vi "Process.vi"(8 "error in":errorcluster, 11 "Inst.Attocube-3DR":refnum<class "Inst.Attocube-3DR.lvclass">) -> (0 "error out":errorcluster, 3 "Inst.Attocube-3DR out":refnum<class "Inst.Attocube-3DR.lvclass">)   [LabVIEW 2019, in "Inst.Attocube-3DR.lvclass"]
doc: "---------------------------------------------------------------\nJKI State Machine Objects™\nhttp://jki.net/state-machine-objects/\nCopyright (C) 2005-2015, JKI <info@jki.net>\nALL RIGHTS RESERVED"
uses:
  Inst.Attocube-3DR.lvclass
  <vilib>/JKI/JKI SMO/SMO/SMO.lvclass
  <userlib>/LevyLab/Instrument Framework/SMOs/Instrument/Instrument.lvclass
  C:/Program Files (x86)/National Instruments/LabVIEW 2019/user.lib/LevyLab/Instrument Framework/Instrument Types/VSource/Instrument.VSource.lvclass
  C:/Program Files (x86)/National Instruments/LabVIEW 2019/user.lib/LevyLab/Instrument Framework/SMOs/Instrument/Instrument.lvclass
  C:/Program Files (x86)/National Instruments/LabVIEW 2019/vi.lib/JKI/JKI SMO/SMO/SMO.lvclass
  <userlib>/LevyLab/Instrument Framework/SMOs/RemoteControl/Typedefs/Message--Cluster.ctl
  <userlib>/LevyLab/Instrument Framework/SMOs/RemoteControl/RemoteControl.lvclass
  Typedefs/PrivateEvents--Inst.Attocube-3DR.MessageToProcess.ctl
  <userlib>/LevyLab/Instrument Framework/Instrument Types/VSource/Instrument.VSource.lvclass
  02efe66c-2260-4f62-810d-420fe48266f6.vi
  Typedefs/Inst.Attocube-3DR.Inputs--Cluster.ctl
  b2d5f30b-306e-4431-881a-eae28691b89f.vi
  0d401355-90ab-4fe7-b69d-5d5dba6cf2d1.vi
  f6063e37-5151-4c3e-a0a1-ff20a9429030.vi
  b7011c9a-a6eb-4fed-9c65-84cbf090edec.vi
  a7b2e31e-1869-440d-b8a6-16844ca516c9.vi
  646a4127-2411-415a-a65c-d25643f6d308.vi
  9e0d4248-952c-4312-a65b-c2252510a20b.vi
  91b4fc71-810e-4ac6-861b-a834e2ae1df3.vi
  7463a076-c03a-4db0-a820-c31f80c245ec.vi
  b30ad2a8-5df5-4a5a-98b2-da7e262b1587.vi
  0967008a-f394-440b-b6da-68de688ceb32.vi
  53937d0e-537d-4a87-94d7-f09408c92319.vi
  61d2fe89-1505-4e67-8cee-d03c7fbfaeb2.vi
panel:
  out "Status":string
  out "State History":string
  # "Instrument.Framework-Template"
  # "Framework-Template"
  # "For instructions on how to use the JKI State Machine Objects, examples and video tutorials, visit:\nhttp://jki.net/state-machine-objects/\n\nJKI State Machine Objects™\nhttp://jki.net/state-machine-objects/\nCopyright (C) 2005-2015, JKI <info@jki.net>\nALL RIGHTS RESERVED"
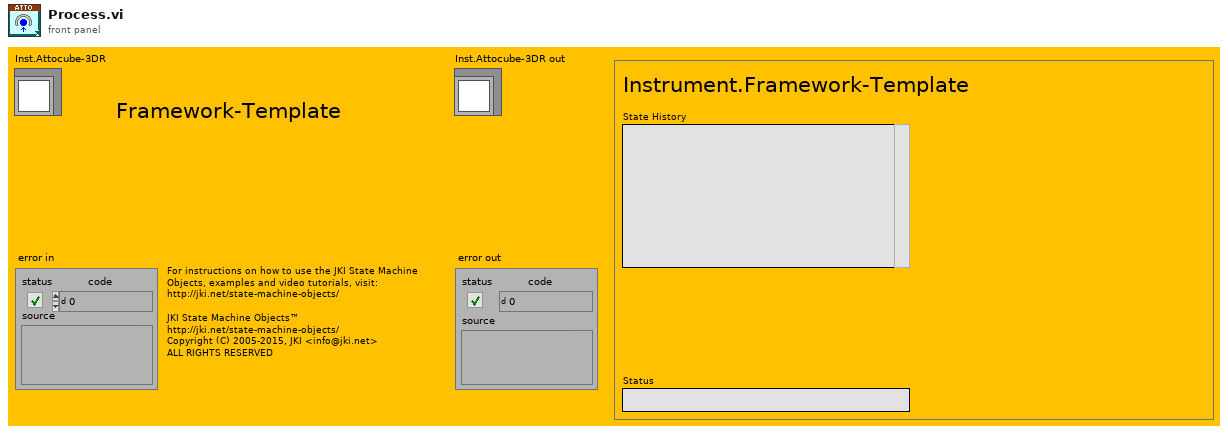
[diagram p1: front panel]
types:
  T1 = enum32{"invalid app kind", "Development System", "Run Time System", "Student Edition", "Embedded LabVIEW", "Evaluation", "Custom"}
  T2 = enum32{"Invalid", "Standard", "Closed", "Hidden", "Minimized", "Maximized"}
  T3 = typedef "RemoteControl.lvclass/Message--Cluster.ctl" = cluster{"Command":string, "Data":variant, "ID":string}
  T4 = typedef "Inst.Attocube-3DR.lvclass/PrivateEvents--Inst.Attocube-3DR.MessageToProcess.ctl" = cluster{"Message":T3}
  T5 = cluster{"Core":cluster{"Current VI Reference":refnum<vi>, "Close Panel on Exit?":bool, "Last Error":cluster{"error":errorcluster, "previous state":string, "remaining states":string}, "Shutdown?":bool}, "SelfRef":refnum<class "Inst.Attocube-3DR.lvclass">, "Running Step":i32, "sequence":string[], "MessageToProcess":T4}
  T6 = cluster{"Current VI Reference":refnum<vi>, "Close Panel on Exit?":bool, "Last Error":cluster{"error":errorcluster, "previous state":string, "remaining states":string}, "Shutdown?":bool}
  T7 = typedef "SMO.lvclass/Protected Events.ctl" = cluster{"StopProcesses":refnum<user-event>, "AbortProcesses":refnum<user-event>, "Config Changed":refnum<user-event>, "Dependency":refnum<user-event>}
  T8 = typedef "Inst.Attocube-3DR.lvclass/Inst.Attocube-3DR.Inputs--Cluster.ctl" = cluster{"Handle":i32, "Axes Number":u8, "Axis 1: sp Position":dbl, "Axis 2: sp Position":dbl, "Axis 1: sp rot count":i32, "Axis 2: sp rot count":i32, "Backward or Forward?":bool, "Axis 1: Amplitude [V] ":dbl, "Axis 2: Amplitude [V] ":dbl, "Axis 1: DCLevel [V]":dbl, "Axis 2: DCLevel [V]":dbl, "Axis 1: Frequency [Hz]":i32, "Axis 2: Frequency [Hz]":i32, "Axis 1:\ncontrol mode":enum16{"speed", "amplitude", "step size"}, "Axis 2:\ncontrol mode":enum16{"speed", "amplitude", "step size"}, "axis 1:\nOutput":bool, "axis 2:\nOutput 2":bool, "axis 1:\nstop detection":bool, "axis 2:\nstop detection":bool, "axis 1:\nSingle Circle Mode":bool, "axis 2:\nSingle Circle Mode":bool, "axis 1: \nTarget GND":bool, "axis 2: \nTarget GND":bool}
  T9 = cluster{"error ":bool, "error number":i32, "error code":string}
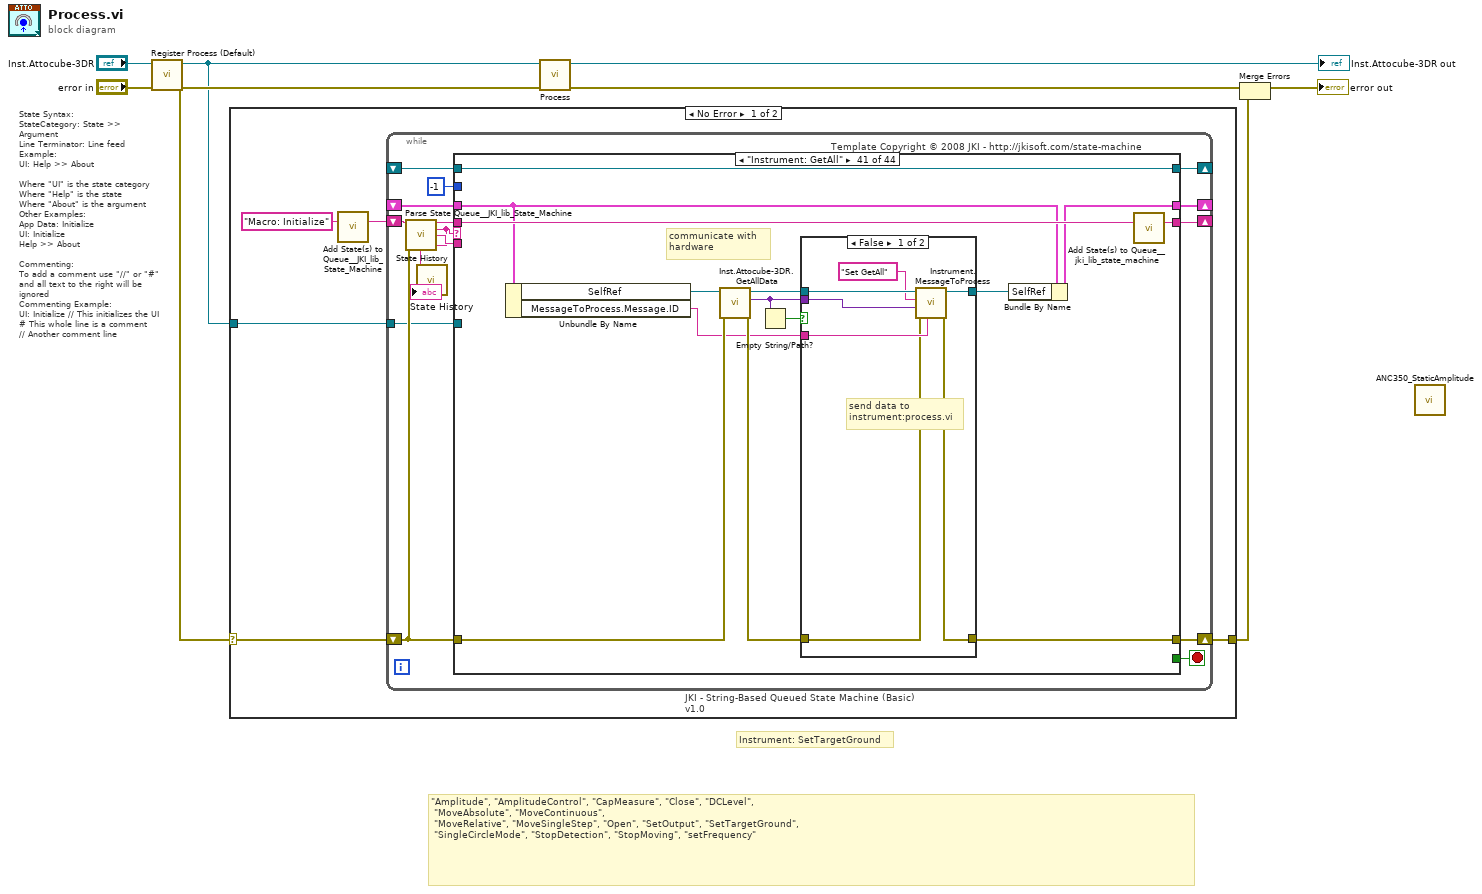
[diagram p0: block diagram]
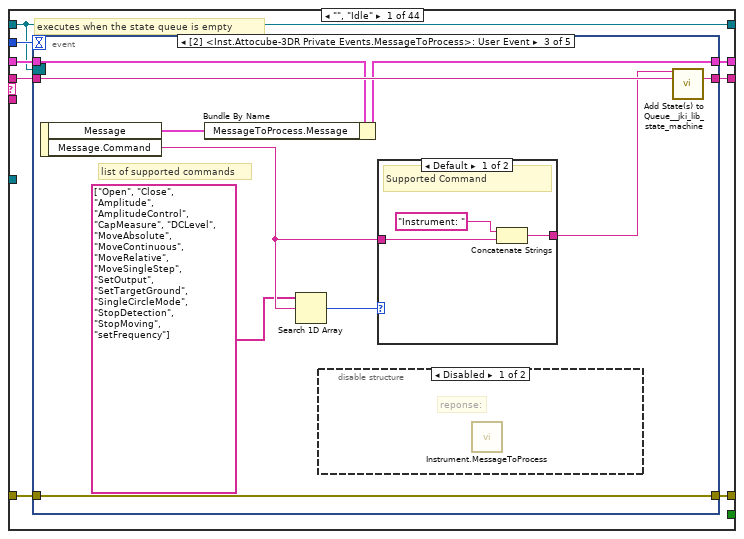
[diagram p2: hidden frame]
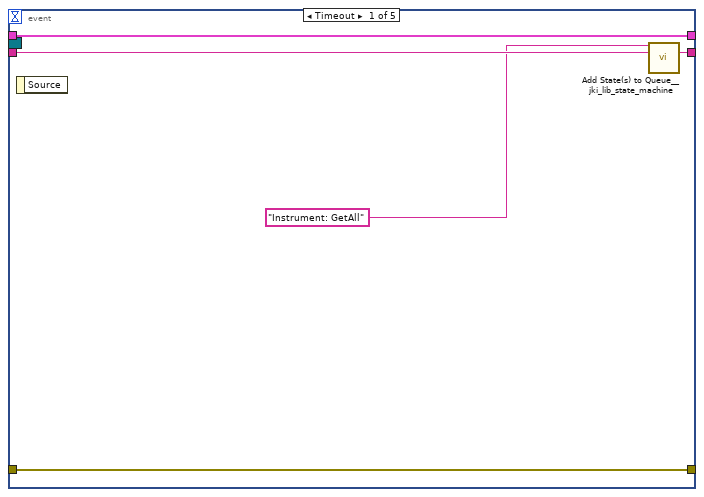
[diagram p3: hidden frame]
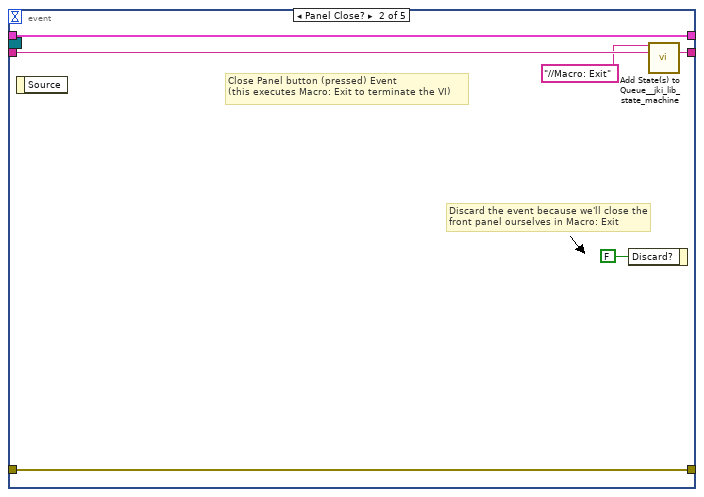
[diagram p4: hidden frame]
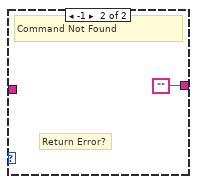
[diagram p6: hidden frame]
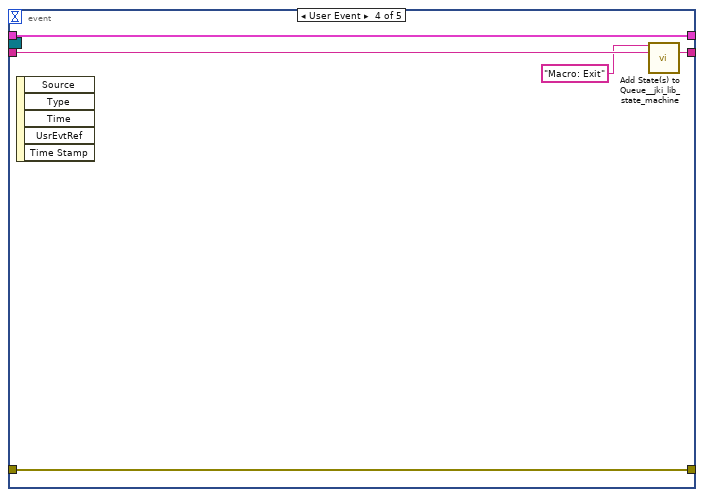
[diagram p7: hidden frame]
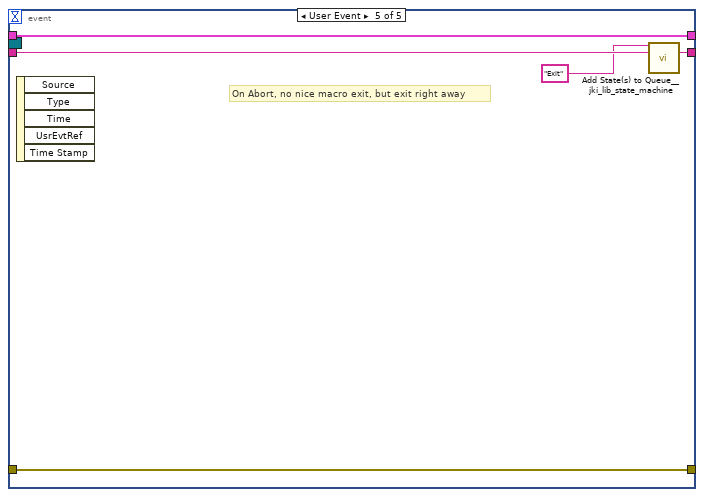
[diagram p8: hidden frame]
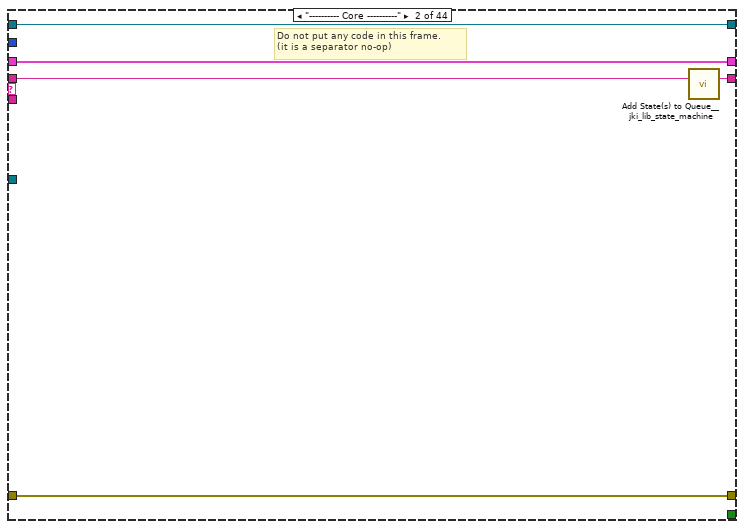
[diagram p9: hidden frame]
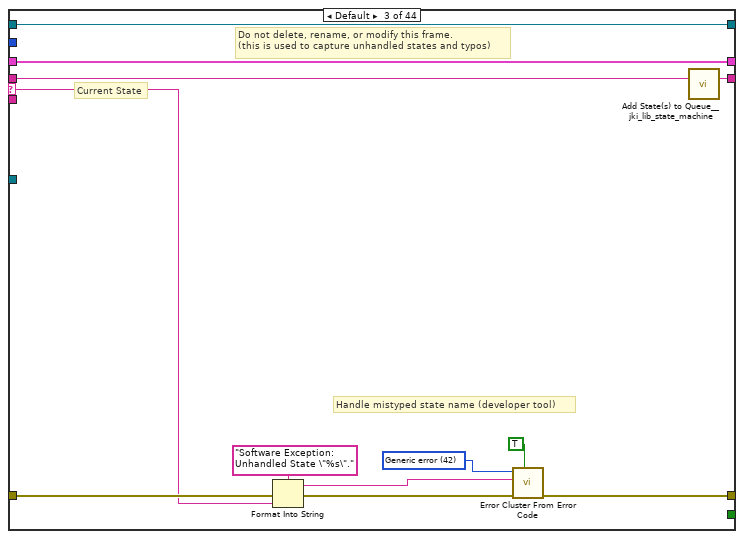
[diagram p10: hidden frame]
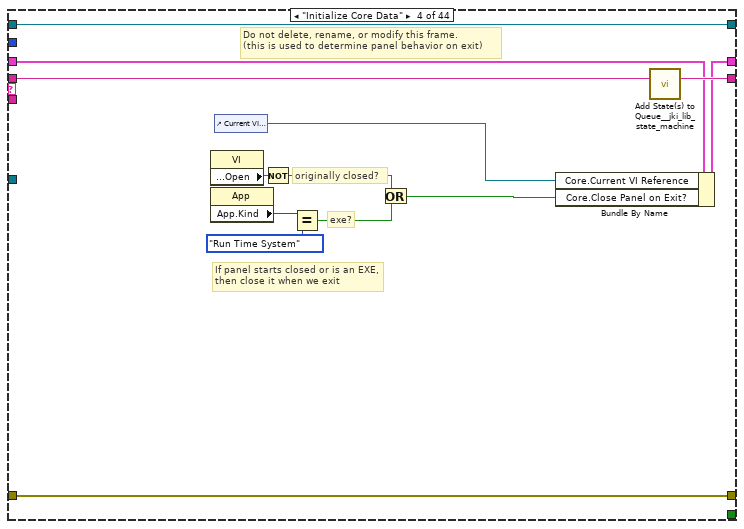
[diagram p11: hidden frame]
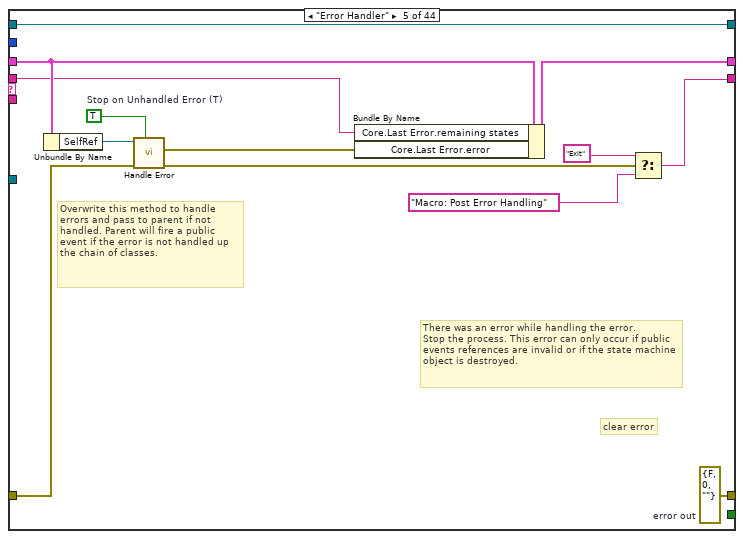
[diagram p12: hidden frame]
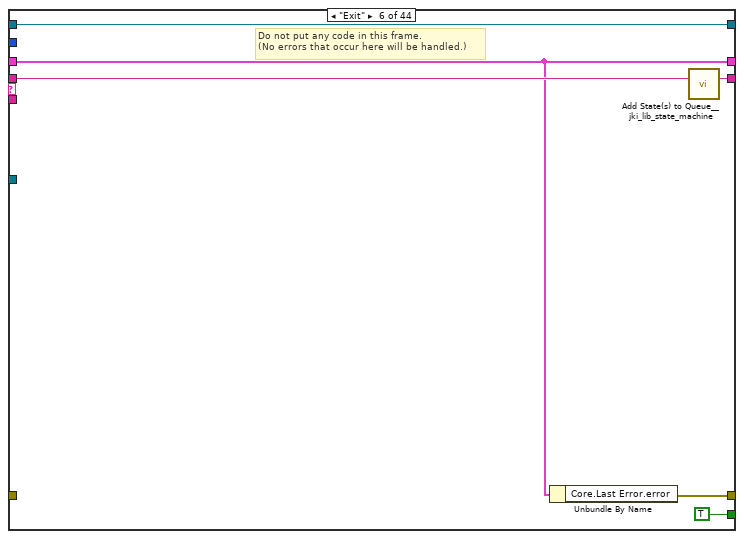
[diagram p13: hidden frame]
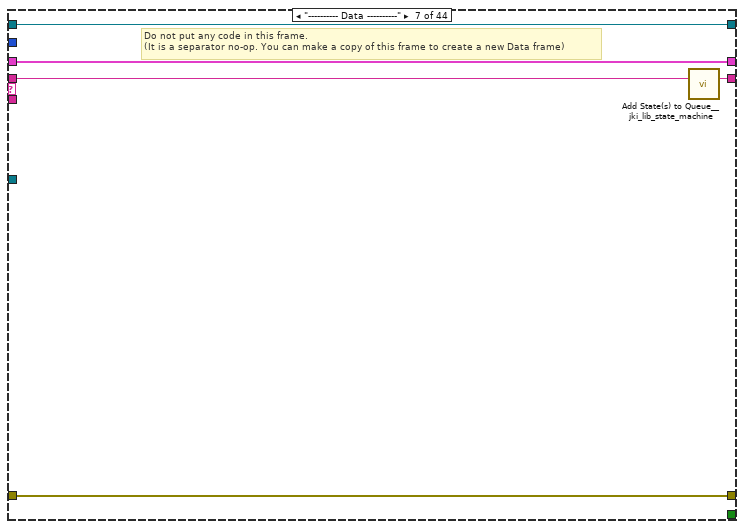
[diagram p14: hidden frame]
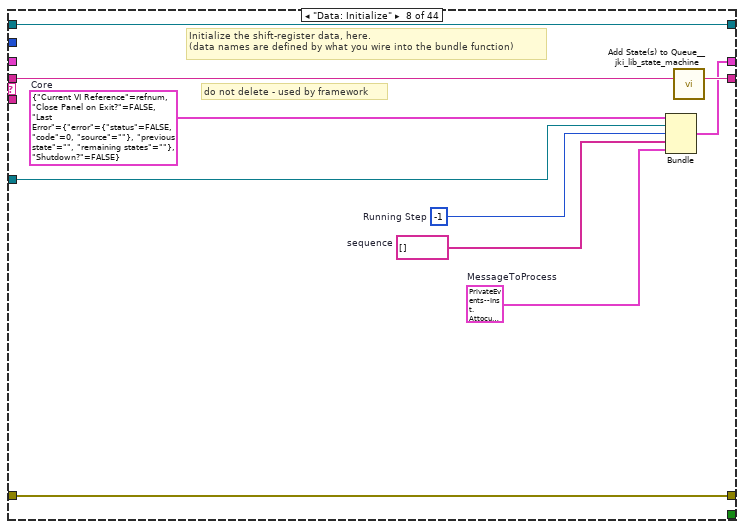
[diagram p15: hidden frame]
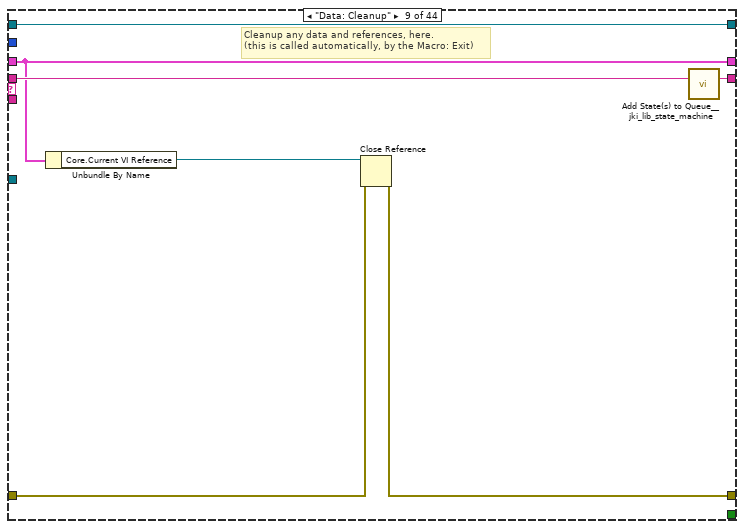
[diagram p16: hidden frame]
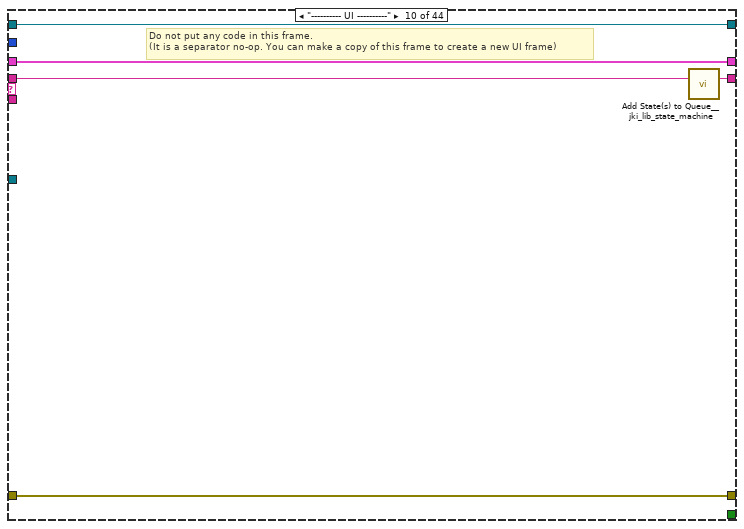
[diagram p17: hidden frame]
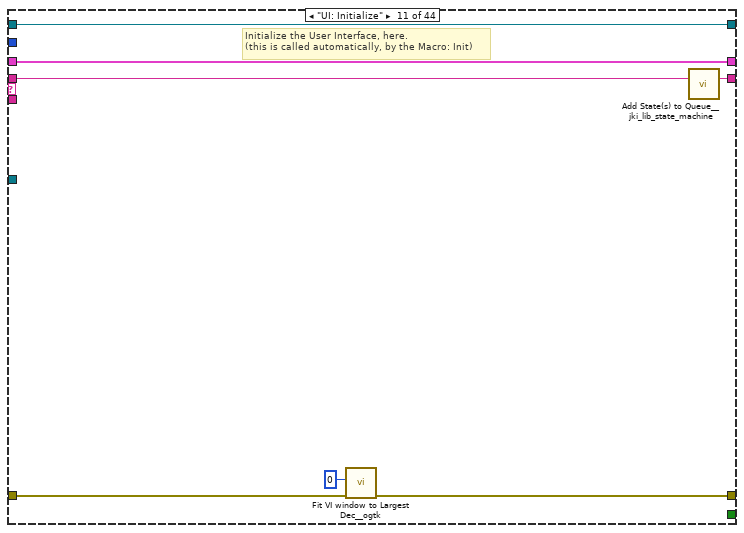
[diagram p18: hidden frame]
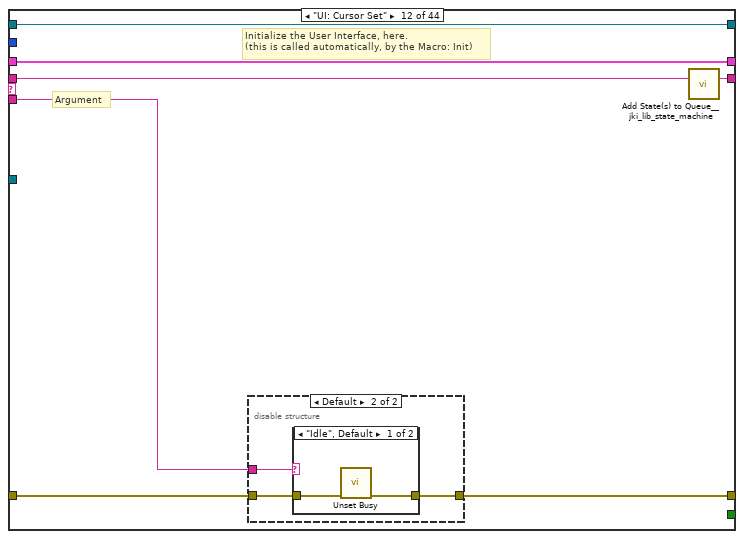
[diagram p19: hidden frame]
diagram:
  # "Instrument: SetTargetGround"
  # "\"Amplitude\", \"AmplitudeControl\", \"CapMeasure\", \"Close\", \"DCLevel\",\n \"MoveAbsolute\", \"MoveContinuous\",\n \"MoveRelative\", \"MoveSingleStep\", \"Open\", \"SetOutput\", \"SetTargetGround\",\n \"SingleCircleMode\", \"StopDetection\", \"StopMoving\", \"setFrequency\""
  # "State Syntax:\nStateCategory: State >> Argument\nLine Terminator: Line feed\nExample:\nUI: Help >> About\n\nWhere \"UI\" is the state category\nWhere \"Help\" is the state\nWhere \"About\" is the argument\nOther Examples:\nApp Data: Initialize\nUI: Initialize\nHelp >> About\n\nCommenting:\nTo add a comment use \"//\" or \"#\" and all text to the right will be ignored\nCommenting Example:\nUI: Initialize // This initializes the UI\n# This whole line is a comment\n// Another comment line"
  n1 = call <vilib>:"Register Process (Default).vi"("error in (no error)"="error in", "SMO"="Inst.Attocube-3DR") -> ("error out"=w5:errorcluster, "SelfRef"=w4:refnum<class "Inst.Attocube-3DR.lvclass">)  [unwired: 8 in]
  n2 = case shown="No Error" w5 {
    selector: w5 -> [w10 w732]
    tunnel: w4 -> [w11 _]
    tunnel: [w9 w732] -> w1
    frame No Error {
      n3 = call <vilib>:"Add State(s) to Queue__JKI_lib_State_Machine.vi"("State(s) in (\"\")"="Macro: Initialize") -> ("States Out"=w13:string)  [unwired: 14 in]
      n4 = while "JKI - String-Based Queued State Machine (Basic) v1.0" {
        shift-right: [w22] -> _
        shift-left: _ -> [w21]
        shift-right: [w25] -> w9
        shift-left: w10 -> [w19]
        shift-right: [w24] -> _
        shift-left: w13 -> [w26]
        tunnel: w11 -> [w18]
        shift-right: [w17] -> _
        shift-left: _ -> [w16]
        stop <- w23 stop-if-true
        # "Template Copyright © 2008 JKI - http://jkisoft.com/state-machine"
        n5 = call <vilib>:"Parse State Queue__JKI_lib_State_Machine.vi"("State Queue"=w26, "Error In (no error)"=w19) -> ("Remaining States"=w28:string, "Current State"=w15:string, "Arguments"=w27:string)  [unwired: 11 in]
        n6 = call <userlib>:"State History.vi"("Current State"=w15) -> ("History"=→"State History":string)  [unwired: 10 in]
        n7 = case shown="\"Instrument: GetAll\"" w15 {
          selector: w15 -> [_ _ w78 _ _ _ _ _ _ _ _ _ _ _ _ _ _ _ _ _ _ _ _ _ _ _ _ _ _ _ _ _ _ _ _ _ _ _ _ _ _ _ _ _]
          tunnel: w28 -> [w36 w76 w82 w101 w106 w120 w125 w135 w142 w147 w154 w161 w177 w209 w228 w240 w261 w283 w288 w299 w304 w317 w323 w330 w347 w369 w390 w413 w436 w459 w482 w505 w529 w555 w581 w608 w631 w654 w669 w678 w692 w706 w712 w731]
          tunnel: w27 -> [_ _ _ _ _ _ _ _ _ _ _ w155 w171 _ _ _ _ _ _ _ _ _ _ _ _ _ _ _ _ _ _ _ _ _ _ _ _ _ _ _ _ _ w707 w715]
          tunnel: w21 -> [w34 w73 w80 w92 w110 w116 w122 _ w137 w144 w152 w159 w173 w206 w225 w230 w251 w264 w285 w296 w301 w310 w321 w325 w343 w365 w386 w409 w432 w455 w478 w501 w525 w551 w577 w604 w627 w650 w665 w674 w680 w702 w708 w721]
          tunnel: [w33 w74 w84 w98 w111 w115 w123 w127 w138 w145 w149 w156 w174 w207 w213 w238 w259 w266 w286 w290 w302 w313 w319 w327 w332 w355 w374 w399 w420 w443 w470 w493 w513 w538 w566 w593 w615 w641 w662 w671 w685 w703 w709 w723] -> w25
          tunnel: w19 -> [w32 w74 w83 w98 w112 _ w123 w127 w139 w145 w148 w157 w175 w207 w217 w238 w259 w267 w286 w291 w302 w307 w319 w327 w333 w356 w375 w400 w421 w444 w469 w492 w514 w539 w567 w594 w616 w642 w661 w670 w688 w703 w709 w717]
          tunnel: [w35 w75 w81 w100 w102 w119 w124 w134 w141 w146 w153 w160 w176 w208 w227 w239 w260 w282 w287 w298 w303 w316 w322 w329 w346 w368 w389 w412 w435 w458 w481 w504 w528 w554 w580 w607 w630 w653 w668 w677 w691 w705 w711 w730] -> w24
          tunnel: [_ _ _ _ _ TRUE _ _ _ _ _ _ _ _ _ _ _ _ _ _ _ _ _ _ _ _ _ _ _ _ _ _ _ _ _ _ _ _ _ _ _ _ _ _] -> w23
          tunnel: [w31 w73 w80 w99 w109 w116 w122 w133 w137 w144 w152 w159 w173 w206 w225 w231 w252 w264 w285 w296 w301 w310 w321 w326 w344 w366 w387 w410 w433 w456 w479 w502 w526 w552 w578 w605 w628 w651 w666 w675 w689 w702 w708 w720] -> w22
          tunnel: -1 ("Timeout") -> [w30 _ _ _ _ _ _ _ _ _ _ _ _ _ _ _ _ _ _ _ _ _ _ _ _ _ _ _ _ _ _ _ _ _ _ _ _ _ _ _ _ _ _ _]
          tunnel: w18 -> [_ _ _ _ _ _ _ w128 _ _ _ _ _ _ w221 _ _ w263 _ _ _ _ _ _ _ _ _ _ _ _ _ _ _ _ _ _ _ _ _ _ _ _ _ _]
          tunnel: [w29 w72 w77 w89 w114 w117 w121 w132 w136 w143 w151 w158 w170 w205 w226 w237 w258 w277 w284 w297 w300 w315 w320 w328 w345 w367 w388 w411 w434 w457 w480 w503 w527 w553 w579 w606 w629 w652 w667 w676 w690 w704 w710 w729] -> w17
          tunnel: w16 -> [w29 w72 w77 w89 w114 w117 w121 w132 w136 w143 w151 w158 w170 w205 w226 w237 w258 w277 w284 w297 w300 _ w320 w328 w345 w367 w388 w411 w434 w457 w480 w503 w527 w553 w579 w606 w629 w652 w667 w676 w690 w704 w710 w729]
          frame "", "Idle" {
            # "executes when the state queue is empty"
            n8 = event shown="[2] <Inst.Attocube-3DR Private Events.MessageToProcess>: User Event" {
              selector: w29 -> [_ _ _ _ _]
              dyn-events: _ -> [_ _ _ _ _]
              timeout: w30 -> [_ _ _ _ _]
              tunnel: w36 -> [w41 w47 w57 w66 w71]
              tunnel: [w40 w46 w56 w65 w70] -> w35
              tunnel: w34 -> [w38 w44 w50 w63 w68]
              tunnel: [w39 w45 w55 w64 w69] -> w33
              tunnel: w32 -> [w39 w45 w55 w64 w69]
              tunnel: [w38 w44 w51 w63 w68] -> w31
              event Timeout {
                n9 = event-data() -> ()  [unwired: 1 in, 1 out]
                n10 = call <vilib>:"Add State(s) to Queue__jki_lib_state_machine.vi"("State(s) in Front (\"\")"="Instrument: GetAll" ("State(s) in Front (\"\")"), "State(s) in (\"\")"=w41) -> ("States Out"=w40:string)  [unwired: 13 in]
              }
              event Panel Close? {
                # "Discard the event because we'll close the front panel ourselves in Macro: Exit"
                # "Close Panel button (pressed) Event\n(this executes Macro: Exit to terminate the VI)"
                n11 = event-data() -> ()  [unwired: 1 in, 1 out]
                n12 = event-data("Discard?"=FALSE) -> ()  [unwired: 1 in, 1 out]
                n13 = call <vilib>:"Add State(s) to Queue__jki_lib_state_machine.vi"("State(s) in Front (\"\")"="//Macro: Exit", "State(s) in (\"\")"=w47) -> ("States Out"=w46:string)  [unwired: 13 in]
              }
              event User Event {
                # "list of supported commands"
                n14 = event-data() -> ("Message"=w49:T3, "Message.Command"=w52:string)  [unwired: 1 in]
                n15 = Bundle By Name(cluster=w50, "MessageToProcess.Message"=w49) -> (w51:T5)
                n16 = Search 1D Array(1D array=string[] ["Open", "Close", "Amplitude", "AmplitudeControl", "CapMeasure", "DCLevel", "MoveAbsolute", "MoveContinuous", "MoveRelative", "MoveSingleStep", "SetOutput", "SetTargetGround", "SingleCircleMode", "StopDetection", "StopMoving", "setFrequency"], element=w52) -> (index of element=w54:i32)  [unwired: 1 in]
                n17 = disable-structure shown="Disabled" {
                  frame Disabled {
                    # "reponse:"
                    n18 = call <userlib>:"Instrument.MessageToProcess.vi"() -> ()  [unwired: 10 in, 2 out]
                  }
                  frame Enabled {
                  }
                }
                n19 = case shown="Default" w54 {
                  tunnel: [w60 "" ("Empty String Constant")] -> w53
                  tunnel: w52 -> [w59 _]
                  frame Default {
                    # "Supported Command"
                    n20 = Concatenate Strings("Instrument: ", w59) -> (w60:string)
                  }
                  frame -1 {
                    # "Return Error?"
                    # "Command Not Found"
                  }
                }
                n21 = call <vilib>:"Add State(s) to Queue__jki_lib_state_machine.vi"("State(s) in Front (\"\")"=w53, "State(s) in (\"\")"=w57) -> ("States Out"=w56:string)  [unwired: 13 in]
              }
              event User Event {
                n22 = event-data() -> ()  [unwired: 1 in, 5 out]
                n23 = call <vilib>:"Add State(s) to Queue__jki_lib_state_machine.vi"("State(s) in Front (\"\")"="Macro: Exit", "State(s) in (\"\")"=w66) -> ("States Out"=w65:string)  [unwired: 13 in]
              }
              event User Event {
                # "On Abort, no nice macro exit, but exit right away"
                n24 = event-data() -> ()  [unwired: 1 in, 5 out]
                n25 = call <vilib>:"Add State(s) to Queue__jki_lib_state_machine.vi"("State(s) in Front (\"\")"="Exit", "State(s) in (\"\")"=w71) -> ("States Out"=w70:string)  [unwired: 13 in]
              }
            }
          }
          frame "---------- Core ----------" {
            # "Do not put any code in this frame.\n(it is a separator no-op)"
            n26 = call <vilib>:"Add State(s) to Queue__jki_lib_state_machine.vi"("State(s) in (\"\")"=w76) -> ("States Out"=w75:string)  [unwired: 14 in]
          }
          frame Default {
            w87 = 42 items=["No error", "Argument error", "Memory is full", "Out of zone", "End of file", "File already open", "Generic file I/O error", "File not found", "File permission error", "Disk is full", "Duplicate path", "Too many files open", "System feature not enabled", "Resource file not found", "Cannot add resource", "Resource not found", "Image not found", "Image memory error", "Pen does not exist", "Config type invalid", "Config token not found", "Config parse error", "Config memory error", "Bad external code format", "Bad external code offset", "External code not present", "Null window", "Destroy window error", "Null menu", "Print aborted", "Bad print record", "Print driver error", "Windows error during printing", "Memory error during printing", "Print dialog error", "Generic print error", "Invalid device refnum", "Device not found", "Device parameter error", "Device unit error", "Cannot open device", "Device call aborted", "Generic error", "Cancelled by user", "Object ID too low", "Object ID too high", "Object not in heap", "Unknown heap", "Unknown object (invalid DefProc)", "Unknown object (DefProc not in table)", "Message out of range", "Invalid (null) method", "Unknown message", "Manager call not supported", "Bad address", "Network operation in progress", "Network operation timed out", "Connection is busy", "Network attribute not supported", "Network error", "Address in use", "System out of memory", "Connection aborted", "Connection refused", "Not connected", "Already connected", "Connection closed", "Initialization error (interapplication manager)", "Bad occurrence", "Wait on unbound occurrence handler", "Occurrence queue overflow", "Datalog type conflict", "Unused", "Unrecognized type (interapplication manager)", "Memory corrupt", "Failed to make temporary DLL", "Old CIN version", "Drag socket not found", "Failed to load drop-object", "Failed to register OLE object", "Failed to release OLE object", "Format specifier type mismatch", "Unknown format specifier", "Too few format specifiers", "Too many format specifiers", "Scan failed", "Newer CIN version", "Error converting to variant", "Runtime menu error", "Password tampered", "Variant attribute not found", "Incompatible variant data type", "Event data is not available", "Event Store is not present", "Occurrence is not found", "Event Queue is not created", "Event info is not available", "Refnum passed is NULL", "Error retrieving Class GUID", "Error retrieving CoClass GUID", "Error retrieving TypeLib GUID.", "Bad built application magic bytes.", "Specific driver is different from the specific driver associated with the Logical Name.", "There is no session opened to the class driver.", "Max Error", "MAX - Error with config objects", "MAX - Error loading configuration", "MAX - Group not supported"]
            # "Current State"
            # "Do not delete, rename, or modify this frame.\n(this is used to capture unhandled states and typos)"
            # "Handle mistyped state name (developer tool)"
            n27 = Format Into String(format string="Software Exception: Unhandled State \"%s\"." ("message"), error in=w83, w78) -> (resulting string=w86:string, error out=w85:errorcluster)  [unwired: 1 in]
            n28 = call <vilib>:"Error Cluster From Error Code.vi"("show call chain? (False)"=TRUE, "error in (no error)"=w85, "error message (\"\")"=w86, "error code (0)"=w87) -> ("error out"=w84:errorcluster)  [unwired: 5 in]
            n29 = call <vilib>:"Add State(s) to Queue__jki_lib_state_machine.vi"("State(s) in (\"\")"=w82) -> ("States Out"=w81:string)  [unwired: 14 in]
          }
          frame "Initialize Core Data" {
            # "Do not delete, rename, or modify this frame.\n(this is used to determine panel behavior on exit)"
            # "originally closed?"
            # "exe?"
            # "If panel starts closed or is an EXE, then close it when we exit"
            n30 = property class="VI"() -> ("Front Panel.Open"=w97:bool)  [unwired: 2 in, 2 out]
            n31 = property class="App"() -> ("App.Kind"=w96:T1)  [unwired: 2 in, 2 out]
            n32 = control-ref of="Current VI Reference"() -> (w90:refnum<vi>)
            n33 = Not(x=w97) -> (.not. x?=w94:bool)
            n34 = Equal?(x=w96, y=T1."Run Time System" ("Application:Kind")) -> (x = y?=w93:bool)
            n35 = Or(x=w94, y=w93) -> (x .or. y?=w91:bool)
            n36 = Bundle By Name(cluster=w92, "Core.Current VI Reference"=w90, "Core.Close Panel on Exit?"=w91) -> (w99:T5)
            n37 = call <vilib>:"Add State(s) to Queue__jki_lib_state_machine.vi"("State(s) in (\"\")"=w101) -> ("States Out"=w100:string)  [unwired: 14 in]
          }
          frame "Error Handler" {
            w107 = TRUE  # Stop on Unhandled Error (T)
            w111 = errorcluster {"status"=FALSE, "code"=0, "source"=""}  # error out
            # "clear error"
            # "There was an error while handling the error.\nStop the process. This error can only occur if public events references are invalid or if the state machine object is destroyed."
            # "Overwrite this method to handle errors and pass to parent if not handled. Parent will fire a public event if the error is not handled up the chain of classes."
            n38 = Unbundle By Name(w110) -> ("SelfRef"=w113:refnum<class "Inst.Attocube-3DR.lvclass">)
            n39 = call-dynamic "Handle Error.vi"("Stop on Unhandled Error (T)"=w107, "error in"=w112, "SMO"=w113) -> ("handling error"=w103:errorcluster, "Unhandled error"=w108:errorcluster)  [unwired: 6 in, 1 out]
            n40 = Bundle By Name(cluster=w110, "Core.Last Error.remaining states"=w106, "Core.Last Error.error"=w108) -> (w109:T5)
            n41 = Select(t="Exit", s=w103, f="Macro: Post Error Handling") -> (s? t:f=w102:string)
          }
          frame "Exit" {
            # "Do not put any code in this frame.\n(No errors that occur here will be handled.)"
            n42 = Unbundle By Name(w116) -> ("Core.Last Error.error"=w115:errorcluster)
            n43 = call <vilib>:"Add State(s) to Queue__jki_lib_state_machine.vi"("State(s) in (\"\")"=w120) -> ("States Out"=w119:string)  [unwired: 14 in]
          }
          frame "---------- Data ----------" {
            # "Do not put any code in this frame.\n(It is a separator no-op. You can make a copy of this frame to create a new Data frame)"
            n44 = call <vilib>:"Add State(s) to Queue__jki_lib_state_machine.vi"("State(s) in (\"\")"=w125) -> ("States Out"=w124:string)  [unwired: 14 in]
          }
          frame "Data: Initialize" {
            w126 = T4 {"Message"={"Command"="", "Data"=variant(string ""), "ID"=""}}  # MessageToProcess
            w129 = string[] []  # sequence
            w130 = -1  # Running Step
            w131 = T6 {"Current VI Reference"=refnum, "Close Panel on Exit?"=FALSE, "Last Error"={"error"={"status"=FALSE, "code"=0, "source"=""}, "previous state"="", "remaining states"=""}, "Shutdown?"=FALSE}  # Core
            # "do not delete - used by framework"
            # "Initialize the shift-register data, here.\n(data names are defined by what you wire into the bundle function)"
            n45 = Bundle("Core"=w131, "SelfRef"=w128, "Running Step"=w130, "sequence"=w129, "MessageToProcess"=w126) -> (w133:T5)  [unwired: 1 in]
            n46 = call <vilib>:"Add State(s) to Queue__jki_lib_state_machine.vi"("State(s) in (\"\")"=w135) -> ("States Out"=w134:string)  [unwired: 14 in]
          }
          frame "Data: Cleanup" {
            # "Cleanup any data and references, here.\n(this is called automatically, by the Macro: Exit)"
            n47 = Unbundle By Name(w137) -> ("Core.Current VI Reference"=w140:refnum<vi>)
            n48 = Close Reference(reference=w140, error in (no error)=w139) -> (error out=w138:errorcluster)
            n49 = call <vilib>:"Add State(s) to Queue__jki_lib_state_machine.vi"("State(s) in (\"\")"=w142) -> ("States Out"=w141:string)  [unwired: 14 in]
          }
          frame "---------- UI ----------" {
            # "Do not put any code in this frame.\n(It is a separator no-op. You can make a copy of this frame to create a new UI frame)"
            n50 = call <vilib>:"Add State(s) to Queue__jki_lib_state_machine.vi"("State(s) in (\"\")"=w147) -> ("States Out"=w146:string)  [unwired: 14 in]
          }
          frame "UI: Initialize" {
            # "Initialize the User Interface, here.\n(this is called automatically, by the Macro: Init)"
            n51 = call <userlib>:"Fit VI window to Largest Dec__ogtk.vi"("error in (no error)"=w148, "border spacing (2 px)"=0) -> ("error out"=w149:errorcluster)  [unwired: 4 in, 1 out]
            n52 = call <vilib>:"Add State(s) to Queue__jki_lib_state_machine.vi"("State(s) in (\"\")"=w154) -> ("States Out"=w153:string)  [unwired: 14 in]
          }
          frame "UI: Cursor Set" {
            # "Argument"
            # "Initialize the User Interface, here.\n(this is called automatically, by the Macro: Init)"
            n53 = disable-structure shown="Default" {
              disable-tunnel: w157 -> [w162 w165]
              disable-tunnel: [w162 w164] -> w156
              disable-tunnel: w155 -> [_ w163]
              frame condition #0 {
              }
              frame condition #1 (active) {
                n54 = case shown="\"Idle\", Default" w163 {
                  tunnel: w165 -> [w167 w169]
                  tunnel: [w166 w168] -> w164
                  frame "Idle", Default {
                    n55 = call <vilib>:"Unset Busy.vi"("error in (no error)"=w167) -> ("error out"=w166:errorcluster)  [unwired: 10 in]
                  }
                  frame "Busy" {
                    n56 = call <vilib>:"Set Busy.vi"("error in (no error)"=w169) -> ("error out"=w168:errorcluster)  [unwired: 9 in, 1 out]
                  }
                }
              }
            }
            n57 = call <vilib>:"Add State(s) to Queue__jki_lib_state_machine.vi"("State(s) in (\"\")"=w161) -> ("States Out"=w160:string)  [unwired: 14 in]
          }
          frame "UI: Front Panel State" {
            # "Argument"
            # "Set Front Panel Open or Closed\n(Usage: \"UI: Front Panel State >> Open|Close\")"
            n58 = Unbundle By Name(w173) -> ("Core.Current VI Reference"=w172:refnum<vi>)
            n59 = disable-structure shown="TARGET_TYPE==RT" {
              disable-tunnel: w175 -> [w181 w204]
              disable-tunnel: [w180 w204] -> w174
              disable-tunnel: w172 -> [w179 _]
              disable-tunnel: w171 -> [w178 _]
              frame condition #0 (active) {
                n60 = case shown="\"Close\"" w178 {
                  tunnel: w181 -> [w185 w198]
                  tunnel: [w187 w199] -> w180
                  tunnel: w179 -> [w186 w196]
                  frame "Open", Default {
                    n61 = property class="VI"(reference=w186, error in=w185) -> (reference out=w183:refnum<vi>, error out=w184:errorcluster, "FP.State"=w182:T2)
                    n62 = case shown="\"Closed\"" w182 {
                      tunnel: [w190 w193] -> w187
                      tunnel: w184 -> [w189 w193]
                      tunnel: w183 -> [w188 _]
                      frame "Closed" {
                        n63 = invoke class="VI" method="FP.Open"(reference=w188, error in=w189, "Activate"=TRUE, "State"=T2."Standard") -> (error out=w190:errorcluster)  [unwired: 1 in, 4 out]
                      }
                      frame Default {
                      }
                    }
                  }
                  frame "Close" {
                    n64 = property class="VI"(reference=w196, error in=w198) -> (reference out=w195:refnum<vi>, error out=w197:errorcluster, "FP.State"=w194:T2)
                    n65 = case shown="Default" w194 {
                      tunnel: [w200 w203] -> w199
                      tunnel: w197 -> [w200 w202]
                      tunnel: w195 -> [_ w201]
                      frame "Invalid", "Closed" {
                      }
                      frame Default {
                        n66 = invoke class="VI" method="FP.Close"(reference=w201, error in=w202) -> (error out=w203:errorcluster)  [unwired: 1 in, 2 out]
                      }
                    }
                  }
                }
              }
              frame condition #1 {
              }
            }
            n67 = call <vilib>:"Add State(s) to Queue__jki_lib_state_machine.vi"("State(s) in (\"\")"=w177) -> ("States Out"=w176:string)  [unwired: 14 in]
          }
          frame "---------- Macro ----------" {
            # "Do not put any code in this frame.\n(It is a separator no-op. You can make a copy of this frame to create a new Macro frame)"
            n68 = call <vilib>:"Add State(s) to Queue__jki_lib_state_machine.vi"("State(s) in (\"\")"=w209) -> ("States Out"=w208:string)  [unwired: 14 in]
          }
          frame "Macro: Initialize" {
            # "Initialization Macro\n(This is called once, when the VI starts)"
            n69 = call-dynamic "Read Debug Mode.vi"("error in (no error)"=w217, "Instrument in"=w221) -> ("error out"=w216:errorcluster, "Debug Mode?"=w218:bool)  [unwired: 7 in, 1 out]
            n70 = call <userlib>:"Wait (ms)__ogtk.vi"("error in (no error)"=w216, "milliseconds to wait"=u32 0) -> ("error out"=w213:errorcluster)  [unwired: 8 in, 1 out]
            n71 = Select(t="Open", s=w218, f="Close") -> (s? t:f=w214:string)
            n72 = Format Into String(format string="UI: Initialize\nUI: Front Panel State >> %s\nInstrument: Open Hardware", initial string="", w214) -> (resulting string=w215:string)  [unwired: 1 in, 1 out]
            n73 = call <vilib>:"Add State(s) to Queue__jki_lib_state_machine.vi"("State(s) in Front (\"\")"="Data: Initialize\nInitialize Core Data\nEvents: Register", "State(s) in (\"\")"="Process: Sync", "State(s) at Back (\"\")"=w215) -> ("States Out"=w223:string)  [unwired: 12 in]
            n74 = call <vilib>:"Add State(s) to Queue__jki_lib_state_machine.vi"("State(s) in Front (\"\")"=w223, "State(s) in (\"\")"=w228) -> ("States Out"=w227:string)  [unwired: 13 in]
          }
          frame "Macro: Post Error Handling" {
            # "Clear Last Error?"
            n75 = Unbundle By Name(w230) -> ("Core.Last Error.remaining states"=w232:string, "Core.Shutdown?"=w233:bool)
            n76 = Unbundle By Name(w230) -> ("Core.Last Error.error"=w236:errorcluster)
            n77 = case shown="False" FALSE {
              tunnel: w236 -> [w244 _]
              tunnel: [w244 _] -> w235
              frame False {
              }
              frame True {
              }
            }
            n78 = case shown="True" w233 {
              tunnel: w232 -> [w241 w243]
              tunnel: [w241 w242] -> w229
              frame False {
                # "These are the remaining states (at the moment the error occured). States can be altered according to business logic."
                # "NOT SHUTTING DOWN"
              }
              frame True {
                # "Developer can decide to alter the states but should be aware that during the shutdown process, there are certain states that must be run for the SMO to properly shut itself (and this process) down. As such, one can add states to perform additional clean-ups, but should append the remaining state to be executed."
                # "SHUTTING DOWN"
                n79 = call <vilib>:"Add State(s) to Queue__jki_lib_state_machine.vi"("State(s) in (\"\")"=w243) -> ("States Out"=w242:string)  [unwired: 14 in]
              }
            }
            n80 = Bundle By Name(cluster=w230, "Core.Last Error.error"=w235) -> (w231:T5)
            n81 = call <vilib>:"Add State(s) to Queue__jki_lib_state_machine.vi"("State(s) in Front (\"\")"=w229, "State(s) in (\"\")"=w240) -> ("States Out"=w239:string)  [unwired: 13 in]
          }
          frame "Macro: Run Sequence" {
            # "0,1,2,3,4,"
            # "5"
            # "Do not put any code in this frame.\n(It is a separator no-op. You can make a copy of this frame to create a new Macro frame)"
            n82 = Unbundle By Name(w251) -> ("sequence"=w247:string[], "Running Step"=w245:i32)
            n83 = Array Size(array=w247) -> (size(s)=w257:i32)
            n84 = Index Array(array=w247, index=w245) -> (element=w246:string)
            n85 = Greater Or Equal?(x=w257, y=w245) -> (x >= y?=w249:bool)
            n86 = Select(t=-1 ("Running Step"), s=w249, f=w245) -> (s? t:f=w256:i32)
            n87 = Bundle By Name(cluster=w251, "Running Step"=w256) -> (w252:T5)
            n88 = Select(t="Sequence: Status >> ...", s=w249, f="Idle //Check Event Structure\nMacro: Run Sequence" ("State(s) at Back (\"\")")) -> (s? t:f=w248:string)
            n89 = call <vilib>:"Add State(s) to Queue__jki_lib_state_machine.vi"("State(s) in Front (\"\")"=w246, "State(s) at Back (\"\")"=w248) -> ("States Out"=w250:string)  [unwired: 13 in]
            n90 = call <vilib>:"Add State(s) to Queue__jki_lib_state_machine.vi"("State(s) in Front (\"\")"=w250, "State(s) in (\"\")"=w261) -> ("States Out"=w260:string)  [unwired: 13 in]
          }
          frame "Macro: Exit" {
            # "Exit Macro\n(This is called once, when the VI exits)"
            n91 = Unbundle By Name(w264) -> ("Core.Close Panel on Exit?"=w281:bool)
            n92 = call-dynamic "Read Debug Mode.vi"("error in (no error)"=w267, "Instrument in"=w263) -> ("error out"=w266:errorcluster, "Debug Mode?"=w265:bool)  [unwired: 7 in, 1 out]
            n93 = Select(t="Open", s=w265, f="Close") -> (s? t:f=w271:string)
            n94 = call <vilib>:"Build State String with Arguments__JKI_lib_State_Machine.vi"("Arguments (\"\")"=w271, "State"="UI: Front Panel State") -> ("State with Arguments"=w268:string)  [unwired: 4 in]
            n95 = Select(t=w268, s=w281, f="" ("Empty String Constant")) -> (s? t:f=w279:string)
            n96 = call <vilib>:"Add State(s) to Queue__jki_lib_state_machine.vi"("State(s) in Front (\"\")"="Data: Cleanup\nEvents: Unregister", "State(s) in (\"\")"="Process: Sync", "State(s) at Back (\"\")"="Exit") -> ("States Out"=w274:string)  [unwired: 12 in]
            n97 = call <vilib>:"Add State(s) to Queue__jki_lib_state_machine.vi"("State(s) in Front (\"\")"="Instrument: Close Hardware", "State(s) in (\"\")"=w279, "State(s) at Back (\"\")"=w274) -> ("States Out"=w278:string)  [unwired: 12 in]
            n98 = call <vilib>:"Add State(s) to Queue__jki_lib_state_machine.vi"("State(s) in Front (\"\")"=w278, "State(s) in (\"\")"=w283) -> ("States Out"=w282:string)  [unwired: 13 in]
          }
          frame "---------- Process ----------" {
            # "Template Separator\n(You can make a copy of, or modify, this frame)"
            n99 = call <vilib>:"Add State(s) to Queue__jki_lib_state_machine.vi"("State(s) in (\"\")"=w288) -> ("States Out"=w287:string)  [unwired: 14 in]
          }
          frame "Process: Sync" {
            n100 = Unbundle By Name(w296) -> ("SelfRef"=w292:refnum<class "Inst.Attocube-3DR.lvclass">)
            n101 = call <vilib>:"WaitOnProcessSync.vi"("error in (no error)"=w291, "SMO"=w292) -> ("error out"=w290:errorcluster, "Don't run?"=w295:bool)  [unwired: 7 in, 1 out]
            n102 = Select(t="Data: Cleanup\nEvents: Unregister\nExit", s=w295, f="" ("Empty String Constant")) -> (s? t:f=w289:string)
            n103 = call <vilib>:"Add State(s) to Queue__jki_lib_state_machine.vi"("State(s) in Front (\"\")"=w289, "State(s) in (\"\")"=w299) -> ("States Out"=w298:string)  [unwired: 13 in]
          }
          frame "---------- Events ----------" {
            # "Template Separator\n(You can make a copy of, or modify, this frame)"
            n104 = call <vilib>:"Add State(s) to Queue__jki_lib_state_machine.vi"("State(s) in (\"\")"=w304) -> ("States Out"=w303:string)  [unwired: 14 in]
          }
          frame "Events: Register" {
            n105 = Unbundle By Name(w310) -> ("SelfRef"=w311:refnum<class "Inst.Attocube-3DR.lvclass">)
            n106 = call <vilib>:"GetProtectedEvents.vi"("SMO"=w311) -> ("error out"=w309:errorcluster, "SMO Protected Events"=w314:T7, "SMO out"=w308:refnum<class "Inst.Attocube-3DR.lvclass">)  [unwired: 8 in]
            n107 = call "Inst.Attocube-3DR.GetPrivateEvents.vi"("Inst.Attocube-3DR in"=w308) -> ("error out"=w305:errorcluster, "Inst.Attocube-3DR Private Events"=w306:cluster{"MessageToProcess":refnum<user-event>})  [unwired: 8 in, 1 out]
            n108 = register-events(w314, w306) -> (reference out=w315:refnum<event-registration>, error out=w312:errorcluster)  [unwired: 2 in]
            n109 = Merge Errors(w312, w305, w309, w307) -> (w313:errorcluster)
            n110 = call <vilib>:"Add State(s) to Queue__jki_lib_state_machine.vi"("State(s) in (\"\")"=w317) -> ("States Out"=w316:string)  [unwired: 14 in]
          }
          frame "Events: Unregister" {
            n111 = Unregister For Events(event registration refnum=w320, error in=w319) -> (error out=w318:errorcluster)
            n112 = call <vilib>:"Clear Errors.vi"("error in (no error)"=w318) -> ()  [unwired: 5 in, 2 out]
            n113 = call <vilib>:"Add State(s) to Queue__jki_lib_state_machine.vi"("State(s) in (\"\")"=w323) -> ("States Out"=w322:string)  [unwired: 14 in]
          }
          frame "---------- Instrument ----------" {
            n114 = Unbundle By Name(w325) -> ("SelfRef"=w324:refnum<class "Inst.Attocube-3DR.lvclass">)
            n115 = Bundle By Name(cluster=w325, "SelfRef"=w324) -> (w326:T5)
            n116 = call <vilib>:"Add State(s) to Queue__jki_lib_state_machine.vi"("State(s) in (\"\")"=w330) -> ("States Out"=w329:string)  [unwired: 14 in]
          }
          frame "Instrument: setFrequency" {
            w341 = T8 {"Handle"=0, "Axes Number"=0, "Axis 1: sp Position"=0.0, "Axis 2: sp Position"=0.0, "Axis 1: sp rot count"=0, "Axis 2: sp rot count"=0, "Backward or Forward?"=FALSE, "Axis 1: Amplitude [V] "=0.0, "Axis 2: Amplitude [V] "=0.0, "Axis 1: DCLevel [V]"=0.0, "Axis 2: DCLevel [V]"=0.0, "Axis 1: Frequency [Hz]"=0, "Axis 2: Frequency [Hz]"=0, "Axis 1:\ncontrol mode"=enum."amplitude", "Axis 2:\ncontrol mode"=enum."amplitude", "axis 1:\nOutput"=FALSE, "axis 2:\nOutput 2"=FALSE, "axis 1:\nstop detection"=FALSE, "axis 2:\nstop detection"=FALSE, "axis 1:\nSingle Circle Mode"=FALSE, "axis 2:\nSingle Circle Mode"=FALSE, "axis 1: \nTarget GND"=FALSE, "axis 2: \nTarget GND"=FALSE}  # Inputs
            n117 = Unbundle By Name(w343) -> ("SelfRef"=w340:refnum<class "Inst.Attocube-3DR.lvclass">, "MessageToProcess.Message.Data"=w342:variant)
            n118 = call "Variant to LV Data.vim"("type"=w341, "JSON Data in"=w342) -> ("Data out"=w338:T8)  [unwired: 6 in, 3 out]
            n119 = Unbundle By Name(w338) -> ("Axes Number"=w337:u8)
            n120 = Equal?(x=w337, y=u8 1) -> (x = y?=w331:bool)
            n121 = Unbundle By Name(w340) -> ("handle"=w336:i32)
            n122 = case shown="True" w331 {
              tunnel: w338 -> [w350 w353]
              tunnel: [w349 w352] -> w335
              tunnel: [w348 w351] -> w334
              frame False {
                n123 = Unbundle By Name(w350) -> ("Axes Number"=w349:u8, "Axis 2: Frequency [Hz]"=w348:i32)
              }
              frame True {
                n124 = Unbundle By Name(w353) -> ("Axes Number"=w352:u8, "Axis 1: Frequency [Hz]"=w351:i32)
              }
            }
            n125 = Bundle By Name(cluster=w343, "SelfRef"=w340) -> (w344:T5)
            n126 = call "ANC350_Frequency.vi"("error in"=w333, "PositionerFrequency [Hz]"=w334, "axis no"=w335, "device handle"=w336) -> ("error out"=w332:T9)  [unwired: 2 in, 1 out]
            n127 = call <vilib>:"Add State(s) to Queue__jki_lib_state_machine.vi"("State(s) in (\"\")"=w347) -> ("States Out"=w346:string)  [unwired: 14 in]
          }
          frame "Instrument: StopMoving" {
            w363 = T8 {"Handle"=0, "Axes Number"=0, "Axis 1: sp Position"=0.0, "Axis 2: sp Position"=0.0, "Axis 1: sp rot count"=0, "Axis 2: sp rot count"=0, "Backward or Forward?"=FALSE, "Axis 1: Amplitude [V] "=0.0, "Axis 2: Amplitude [V] "=0.0, "Axis 1: DCLevel [V]"=0.0, "Axis 2: DCLevel [V]"=0.0, "Axis 1: Frequency [Hz]"=0, "Axis 2: Frequency [Hz]"=0, "Axis 1:\ncontrol mode"=enum."amplitude", "Axis 2:\ncontrol mode"=enum."amplitude", "axis 1:\nOutput"=FALSE, "axis 2:\nOutput 2"=FALSE, "axis 1:\nstop detection"=FALSE, "axis 2:\nstop detection"=FALSE, "axis 1:\nSingle Circle Mode"=FALSE, "axis 2:\nSingle Circle Mode"=FALSE, "axis 1: \nTarget GND"=FALSE, "axis 2: \nTarget GND"=FALSE}  # Inputs
            n128 = Unbundle By Name(w365) -> ("SelfRef"=w362:refnum<class "Inst.Attocube-3DR.lvclass">, "MessageToProcess.Message.Data"=w364:variant)
            n129 = call "Variant to LV Data.vim"("type"=w363, "JSON Data in"=w364) -> ("Data out"=w360:T8)  [unwired: 6 in, 3 out]
            n130 = Unbundle By Name(w360) -> ("Axes Number"=w359:u8)
            n131 = Equal?(x=w359, y=u8 1) -> (x = y?=w358:bool)
            n132 = Unbundle By Name(w362) -> ("handle"=w357:i32)
            n133 = case shown="False" w358 {
              tunnel: w360 -> [w371 w373]
              tunnel: [w370 w372] -> w354
              frame False {
                n134 = Unbundle By Name(w371) -> ("Axes Number"=w370:u8)
              }
              frame True {
                n135 = Unbundle By Name(w373) -> ("Axes Number"=w372:u8)
              }
            }
            n136 = Bundle By Name(cluster=w365, "SelfRef"=w362) -> (w366:T5)
            n137 = call "ANC350_StopMoving.vi"("error in"=w356, "axis no"=w354, "device handle"=w357) -> ("error out"=w355:T9)  [unwired: 3 in, 1 out]
            n138 = call <vilib>:"Add State(s) to Queue__jki_lib_state_machine.vi"("State(s) in (\"\")"=w369) -> ("States Out"=w368:string)  [unwired: 14 in]
          }
          frame "Instrument: SetOutput" {
            w384 = T8 {"Handle"=0, "Axes Number"=0, "Axis 1: sp Position"=0.0, "Axis 2: sp Position"=0.0, "Axis 1: sp rot count"=0, "Axis 2: sp rot count"=0, "Backward or Forward?"=FALSE, "Axis 1: Amplitude [V] "=0.0, "Axis 2: Amplitude [V] "=0.0, "Axis 1: DCLevel [V]"=0.0, "Axis 2: DCLevel [V]"=0.0, "Axis 1: Frequency [Hz]"=0, "Axis 2: Frequency [Hz]"=0, "Axis 1:\ncontrol mode"=enum."amplitude", "Axis 2:\ncontrol mode"=enum."amplitude", "axis 1:\nOutput"=FALSE, "axis 2:\nOutput 2"=FALSE, "axis 1:\nstop detection"=FALSE, "axis 2:\nstop detection"=FALSE, "axis 1:\nSingle Circle Mode"=FALSE, "axis 2:\nSingle Circle Mode"=FALSE, "axis 1: \nTarget GND"=FALSE, "axis 2: \nTarget GND"=FALSE}  # Inputs
            n139 = Unbundle By Name(w386) -> ("SelfRef"=w383:refnum<class "Inst.Attocube-3DR.lvclass">, "MessageToProcess.Message.Data"=w385:variant)
            n140 = call "Variant to LV Data.vim"("type"=w384, "JSON Data in"=w385) -> ("Data out"=w381:T8)  [unwired: 6 in, 3 out]
            n141 = Unbundle By Name(w381) -> ("Axes Number"=w380:u8)
            n142 = Equal?(x=w380, y=u8 1) -> (x = y?=w379:bool)
            n143 = Unbundle By Name(w383) -> ("handle"=w378:i32)
            n144 = case shown="True" w379 {
              tunnel: w381 -> [w393 w396]
              tunnel: [w392 w395] -> w376
              tunnel: [w391 w394] -> w377
              frame False {
                n145 = Unbundle By Name(w393) -> ("Axes Number"=w392:u8, "axis 2:\nOutput 2"=w391:bool)
              }
              frame True {
                n146 = Unbundle By Name(w396) -> ("Axes Number"=w395:u8, "axis 1:\nOutput"=w394:bool)
              }
            }
            n147 = Bundle By Name(cluster=w386, "SelfRef"=w383) -> (w387:T5)
            n148 = call "ANC350_SetOutput.vi"("error in"=w375, "enable"=w377, "axis no"=w376, "device handle"=w378) -> ("error out"=w374:T9)  [unwired: 2 in, 1 out]
            n149 = call <vilib>:"Add State(s) to Queue__jki_lib_state_machine.vi"("State(s) in (\"\")"=w390) -> ("States Out"=w389:string)  [unwired: 14 in]
          }
          frame "Instrument: AmplitudeControl" {
            w407 = T8 {"Handle"=0, "Axes Number"=0, "Axis 1: sp Position"=0.0, "Axis 2: sp Position"=0.0, "Axis 1: sp rot count"=0, "Axis 2: sp rot count"=0, "Backward or Forward?"=FALSE, "Axis 1: Amplitude [V] "=0.0, "Axis 2: Amplitude [V] "=0.0, "Axis 1: DCLevel [V]"=0.0, "Axis 2: DCLevel [V]"=0.0, "Axis 1: Frequency [Hz]"=0, "Axis 2: Frequency [Hz]"=0, "Axis 1:\ncontrol mode"=enum."amplitude", "Axis 2:\ncontrol mode"=enum."amplitude", "axis 1:\nOutput"=FALSE, "axis 2:\nOutput 2"=FALSE, "axis 1:\nstop detection"=FALSE, "axis 2:\nstop detection"=FALSE, "axis 1:\nSingle Circle Mode"=FALSE, "axis 2:\nSingle Circle Mode"=FALSE, "axis 1: \nTarget GND"=FALSE, "axis 2: \nTarget GND"=FALSE}  # Inputs
            n150 = Unbundle By Name(w409) -> ("SelfRef"=w406:refnum<class "Inst.Attocube-3DR.lvclass">, "MessageToProcess.Message.Data"=w408:variant)
            n151 = call "Variant to LV Data.vim"("type"=w407, "JSON Data in"=w408) -> ("Data out"=w397:T8)  [unwired: 6 in, 3 out]
            n152 = Unbundle By Name(w397) -> ("Axes Number"=w404:u8)
            n153 = Equal?(x=w404, y=u8 1) -> (x = y?=w403:bool)
            n154 = Unbundle By Name(w406) -> ("handle"=w402:i32)
            n155 = case shown="True" w403 {
              tunnel: w397 -> [w416 w419]
              tunnel: [w415 w418] -> w401
              tunnel: [w414 w417] -> w398
              frame False {
                n156 = Unbundle By Name(w416) -> ("Axes Number"=w415:u8, "Axis 2:\ncontrol mode"=w414:enum16{"speed", "amplitude", "step size"})
              }
              frame True {
                n157 = Unbundle By Name(w419) -> ("Axes Number"=w418:u8, "Axis 1:\ncontrol mode"=w417:enum16{"speed", "amplitude", "step size"})
              }
            }
            n158 = Bundle By Name(cluster=w409, "SelfRef"=w406) -> (w410:T5)
            n159 = call "ANC350_AmplitudeControl.vi"("error in"=w400, "control mode"=w398, "axis no"=w401, "device handle"=w402) -> ("error out"=w399:T9)  [unwired: 2 in, 1 out]
            n160 = call <vilib>:"Add State(s) to Queue__jki_lib_state_machine.vi"("State(s) in (\"\")"=w413) -> ("States Out"=w412:string)  [unwired: 14 in]
          }
          frame "Instrument: DCLevel" {
            w430 = T8 {"Handle"=0, "Axes Number"=0, "Axis 1: sp Position"=0.0, "Axis 2: sp Position"=0.0, "Axis 1: sp rot count"=0, "Axis 2: sp rot count"=0, "Backward or Forward?"=FALSE, "Axis 1: Amplitude [V] "=0.0, "Axis 2: Amplitude [V] "=0.0, "Axis 1: DCLevel [V]"=0.0, "Axis 2: DCLevel [V]"=0.0, "Axis 1: Frequency [Hz]"=0, "Axis 2: Frequency [Hz]"=0, "Axis 1:\ncontrol mode"=enum."amplitude", "Axis 2:\ncontrol mode"=enum."amplitude", "axis 1:\nOutput"=FALSE, "axis 2:\nOutput 2"=FALSE, "axis 1:\nstop detection"=FALSE, "axis 2:\nstop detection"=FALSE, "axis 1:\nSingle Circle Mode"=FALSE, "axis 2:\nSingle Circle Mode"=FALSE, "axis 1: \nTarget GND"=FALSE, "axis 2: \nTarget GND"=FALSE}  # Inputs
            n161 = Unbundle By Name(w432) -> ("SelfRef"=w429:refnum<class "Inst.Attocube-3DR.lvclass">, "MessageToProcess.Message.Data"=w431:variant)
            n162 = call "Variant to LV Data.vim"("type"=w430, "JSON Data in"=w431) -> ("Data out"=w425:T8)  [unwired: 6 in, 3 out]
            n163 = Unbundle By Name(w425) -> ("Axes Number"=w427:u8)
            n164 = Equal?(x=w427, y=u8 1) -> (x = y?=w426:bool)
            n165 = Unbundle By Name(w429) -> ("handle"=w424:i32)
            n166 = case shown="False" w426 {
              tunnel: w425 -> [w439 w442]
              tunnel: [w438 w441] -> w423
              tunnel: [w437 w440] -> w422
              frame False {
                n167 = Unbundle By Name(w439) -> ("Axes Number"=w438:u8, "Axis 2: DCLevel [V]"=w437:dbl)
              }
              frame True {
                n168 = Unbundle By Name(w442) -> ("Axes Number"=w441:u8, "Axis 1: DCLevel [V]"=w440:dbl)
              }
            }
            n169 = Bundle By Name(cluster=w432, "SelfRef"=w429) -> (w433:T5)
            n170 = call "ANC350_DCLevel.vi"("error in"=w421, "DCLevel [V]"=w422, "axis no"=w423, "device handle"=w424) -> ("error out"=w420:T9)  [unwired: 2 in, 1 out]
            n171 = call <vilib>:"Add State(s) to Queue__jki_lib_state_machine.vi"("State(s) in (\"\")"=w436) -> ("States Out"=w435:string)  [unwired: 14 in]
          }
          frame "Instrument: Amplitude" {
            w453 = T8 {"Handle"=0, "Axes Number"=0, "Axis 1: sp Position"=0.0, "Axis 2: sp Position"=0.0, "Axis 1: sp rot count"=0, "Axis 2: sp rot count"=0, "Backward or Forward?"=FALSE, "Axis 1: Amplitude [V] "=0.0, "Axis 2: Amplitude [V] "=0.0, "Axis 1: DCLevel [V]"=0.0, "Axis 2: DCLevel [V]"=0.0, "Axis 1: Frequency [Hz]"=0, "Axis 2: Frequency [Hz]"=0, "Axis 1:\ncontrol mode"=enum."amplitude", "Axis 2:\ncontrol mode"=enum."amplitude", "axis 1:\nOutput"=FALSE, "axis 2:\nOutput 2"=FALSE, "axis 1:\nstop detection"=FALSE, "axis 2:\nstop detection"=FALSE, "axis 1:\nSingle Circle Mode"=FALSE, "axis 2:\nSingle Circle Mode"=FALSE, "axis 1: \nTarget GND"=FALSE, "axis 2: \nTarget GND"=FALSE}  # Inputs
            n172 = Unbundle By Name(w455) -> ("SelfRef"=w452:refnum<class "Inst.Attocube-3DR.lvclass">, "MessageToProcess.Message.Data"=w454:variant)
            n173 = call "Variant to LV Data.vim"("type"=w453, "JSON Data in"=w454) -> ("Data out"=w448:T8)  [unwired: 6 in, 3 out]
            n174 = Unbundle By Name(w448) -> ("Axes Number"=w450:u8)
            n175 = Equal?(x=w450, y=u8 1) -> (x = y?=w449:bool)
            n176 = Unbundle By Name(w452) -> ("handle"=w447:i32)
            n177 = case shown="True" w449 {
              tunnel: w448 -> [w462 w465]
              tunnel: [w461 w464] -> w446
              tunnel: [w460 w463] -> w445
              frame False {
                n178 = Unbundle By Name(w462) -> ("Axes Number"=w461:u8, "Axis 2: Amplitude [V]"=w460:dbl)
              }
              frame True {
                n179 = Unbundle By Name(w465) -> ("Axes Number"=w464:u8, "Axis 1: Amplitude [V]"=w463:dbl)
              }
            }
            n180 = Bundle By Name(cluster=w455, "SelfRef"=w452) -> (w456:T5)
            n181 = call "ANC350_Amplitude.vi"("error in"=w444, "PositionerAmplitude [V]"=w445, "axis no"=w446, "device handle"=w447) -> ("error out"=w443:T9)  [unwired: 2 in, 1 out]
            n182 = call <vilib>:"Add State(s) to Queue__jki_lib_state_machine.vi"("State(s) in (\"\")"=w459) -> ("States Out"=w458:string)  [unwired: 14 in]
          }
          frame "Instrument: MoveContinuous" {
            w476 = T8 {"Handle"=0, "Axes Number"=0, "Axis 1: sp Position"=0.0, "Axis 2: sp Position"=0.0, "Axis 1: sp rot count"=0, "Axis 2: sp rot count"=0, "Backward or Forward?"=FALSE, "Axis 1: Amplitude [V] "=0.0, "Axis 2: Amplitude [V] "=0.0, "Axis 1: DCLevel [V]"=0.0, "Axis 2: DCLevel [V]"=0.0, "Axis 1: Frequency [Hz]"=0, "Axis 2: Frequency [Hz]"=0, "Axis 1:\ncontrol mode"=enum."amplitude", "Axis 2:\ncontrol mode"=enum."amplitude", "axis 1:\nOutput"=FALSE, "axis 2:\nOutput 2"=FALSE, "axis 1:\nstop detection"=FALSE, "axis 2:\nstop detection"=FALSE, "axis 1:\nSingle Circle Mode"=FALSE, "axis 2:\nSingle Circle Mode"=FALSE, "axis 1: \nTarget GND"=FALSE, "axis 2: \nTarget GND"=FALSE}  # Inputs
            n183 = Unbundle By Name(w478) -> ("SelfRef"=w475:refnum<class "Inst.Attocube-3DR.lvclass">, "MessageToProcess.Message.Data"=w477:variant)
            n184 = call "Variant to LV Data.vim"("type"=w476, "JSON Data in"=w477) -> ("Data out"=w471:T8)  [unwired: 6 in, 3 out]
            n185 = Unbundle By Name(w471) -> ("Axes Number"=w473:u8)
            n186 = Equal?(x=w473, y=u8 1) -> (x = y?=w472:bool)
            n187 = Unbundle By Name(w475) -> ("handle"=w466:i32)
            n188 = case shown="False" w472 {
              tunnel: w471 -> [w485 w488]
              tunnel: [w484 w487] -> w468
              tunnel: [w483 w486] -> w467
              frame False {
                n189 = Unbundle By Name(w485) -> ("Axes Number"=w484:u8, "Backward or Forward?"=w483:bool)
              }
              frame True {
                n190 = Unbundle By Name(w488) -> ("Axes Number"=w487:u8, "Backward or Forward?"=w486:bool)
              }
            }
            n191 = Bundle By Name(cluster=w478, "SelfRef"=w475) -> (w479:T5)
            n192 = call "ANC350_MoveContinuous.vi"("error in"=w469, "step direction"=w467, "axis no"=w468, "device handle"=w466) -> ("error out"=w470:T9)  [unwired: 2 in, 1 out]
            n193 = call <vilib>:"Add State(s) to Queue__jki_lib_state_machine.vi"("State(s) in (\"\")"=w482) -> ("States Out"=w481:string)  [unwired: 14 in]
          }
          frame "Instrument: MoveSingleStep" {
            w499 = T8 {"Handle"=0, "Axes Number"=0, "Axis 1: sp Position"=0.0, "Axis 2: sp Position"=0.0, "Axis 1: sp rot count"=0, "Axis 2: sp rot count"=0, "Backward or Forward?"=FALSE, "Axis 1: Amplitude [V] "=0.0, "Axis 2: Amplitude [V] "=0.0, "Axis 1: DCLevel [V]"=0.0, "Axis 2: DCLevel [V]"=0.0, "Axis 1: Frequency [Hz]"=0, "Axis 2: Frequency [Hz]"=0, "Axis 1:\ncontrol mode"=enum."amplitude", "Axis 2:\ncontrol mode"=enum."amplitude", "axis 1:\nOutput"=FALSE, "axis 2:\nOutput 2"=FALSE, "axis 1:\nstop detection"=FALSE, "axis 2:\nstop detection"=FALSE, "axis 1:\nSingle Circle Mode"=FALSE, "axis 2:\nSingle Circle Mode"=FALSE, "axis 1: \nTarget GND"=FALSE, "axis 2: \nTarget GND"=FALSE}  # Inputs
            n194 = Unbundle By Name(w501) -> ("SelfRef"=w498:refnum<class "Inst.Attocube-3DR.lvclass">, "MessageToProcess.Message.Data"=w500:variant)
            n195 = call "Variant to LV Data.vim"("type"=w499, "JSON Data in"=w500) -> ("Data out"=w494:T8)  [unwired: 6 in, 3 out]
            n196 = Unbundle By Name(w494) -> ("Axes Number"=w496:u8)
            n197 = Equal?(x=w496, y=u8 1) -> (x = y?=w495:bool)
            n198 = Unbundle By Name(w498) -> ("handle"=w489:i32)
            n199 = case shown="True" w495 {
              tunnel: w494 -> [w508 w511]
              tunnel: [w507 w510] -> w490
              tunnel: [w506 w509] -> w491
              frame False {
                n200 = Unbundle By Name(w508) -> ("Axes Number"=w507:u8, "Backward or Forward?"=w506:bool)
              }
              frame True {
                n201 = Unbundle By Name(w511) -> ("Axes Number"=w510:u8, "Backward or Forward?"=w509:bool)
              }
            }
            n202 = Bundle By Name(cluster=w501, "SelfRef"=w498) -> (w502:T5)
            n203 = call "ANC350_MoveSingleStep.vi"("error in"=w492, "single step direction"=w491, "axis no"=w490, "device handle"=w489) -> ("error out"=w493:T9)  [unwired: 2 in, 1 out]
            n204 = call <vilib>:"Add State(s) to Queue__jki_lib_state_machine.vi"("State(s) in (\"\")"=w505) -> ("States Out"=w504:string)  [unwired: 14 in]
          }
          frame "Instrument: MoveRelative" {
            w523 = T8 {"Handle"=0, "Axes Number"=0, "Axis 1: sp Position"=0.0, "Axis 2: sp Position"=0.0, "Axis 1: sp rot count"=0, "Axis 2: sp rot count"=0, "Backward or Forward?"=FALSE, "Axis 1: Amplitude [V] "=0.0, "Axis 2: Amplitude [V] "=0.0, "Axis 1: DCLevel [V]"=0.0, "Axis 2: DCLevel [V]"=0.0, "Axis 1: Frequency [Hz]"=0, "Axis 2: Frequency [Hz]"=0, "Axis 1:\ncontrol mode"=enum."amplitude", "Axis 2:\ncontrol mode"=enum."amplitude", "axis 1:\nOutput"=FALSE, "axis 2:\nOutput 2"=FALSE, "axis 1:\nstop detection"=FALSE, "axis 2:\nstop detection"=FALSE, "axis 1:\nSingle Circle Mode"=FALSE, "axis 2:\nSingle Circle Mode"=FALSE, "axis 1: \nTarget GND"=FALSE, "axis 2: \nTarget GND"=FALSE}  # Inputs
            n205 = Unbundle By Name(w525) -> ("SelfRef"=w522:refnum<class "Inst.Attocube-3DR.lvclass">, "MessageToProcess.Message.Data"=w524:variant)
            n206 = call "Variant to LV Data.vim"("type"=w523, "JSON Data in"=w524) -> ("Data out"=w518:T8)  [unwired: 6 in, 3 out]
            n207 = Unbundle By Name(w518) -> ("Axes Number"=w520:u8)
            n208 = Equal?(x=w520, y=u8 1) -> (x = y?=w519:bool)
            n209 = Unbundle By Name(w522) -> ("handle"=w517:i32)
            n210 = case shown="True" w519 {
              tunnel: w518 -> [w533 w537]
              tunnel: [w532 w536] -> w516
              tunnel: [w531 w535] -> w515
              tunnel: [w530 w534] -> w512
              frame False {
                n211 = Unbundle By Name(w533) -> ("Axes Number"=w532:u8, "Axis 2: sp Position"=w531:dbl, "Axis 2: sp rot count"=w530:i32)
              }
              frame True {
                n212 = Unbundle By Name(w537) -> ("Axes Number"=w536:u8, "Axis 1: sp Position"=w535:dbl, "Axis 1: sp rot count"=w534:i32)
              }
            }
            n213 = Bundle By Name(cluster=w525, "SelfRef"=w522) -> (w526:T5)
            n214 = call "ANC350_MoveRelative.vi"("device handle"=w517, "axis no"=w516, "distance [µm/°/m°]"=w515, "rot count"=w512, "error in"=w514) -> ("error out"=w513:T9)  [unwired: 9 in, 1 out]
            n215 = call <vilib>:"Add State(s) to Queue__jki_lib_state_machine.vi"("State(s) in (\"\")"=w529) -> ("States Out"=w528:string)  [unwired: 14 in]
          }
          frame "Instrument: MoveAbsolute" {
            w549 = T8 {"Handle"=0, "Axes Number"=0, "Axis 1: sp Position"=0.0, "Axis 2: sp Position"=0.0, "Axis 1: sp rot count"=0, "Axis 2: sp rot count"=0, "Backward or Forward?"=FALSE, "Axis 1: Amplitude [V] "=0.0, "Axis 2: Amplitude [V] "=0.0, "Axis 1: DCLevel [V]"=0.0, "Axis 2: DCLevel [V]"=0.0, "Axis 1: Frequency [Hz]"=0, "Axis 2: Frequency [Hz]"=0, "Axis 1:\ncontrol mode"=enum."amplitude", "Axis 2:\ncontrol mode"=enum."amplitude", "axis 1:\nOutput"=FALSE, "axis 2:\nOutput 2"=FALSE, "axis 1:\nstop detection"=FALSE, "axis 2:\nstop detection"=FALSE, "axis 1:\nSingle Circle Mode"=FALSE, "axis 2:\nSingle Circle Mode"=FALSE, "axis 1: \nTarget GND"=FALSE, "axis 2: \nTarget GND"=FALSE}  # Inputs
            n216 = Unbundle By Name(w551) -> ("SelfRef"=w548:refnum<class "Inst.Attocube-3DR.lvclass">, "MessageToProcess.Message.Data"=w550:variant)
            n217 = call "Variant to LV Data.vim"("type"=w549, "JSON Data in"=w550) -> ("Data out"=w544:T8)  [unwired: 6 in, 3 out]
            n218 = Unbundle By Name(w544) -> ("Axes Number"=w546:u8)
            n219 = Equal?(x=w546, y=u8 1) -> (x = y?=w545:bool)
            n220 = Unbundle By Name(w548) -> ("handle"=w543:i32)
            n221 = case shown="True" w545 {
              tunnel: w544 -> [w559 w563]
              tunnel: [w558 w562] -> w542
              tunnel: [w557 w561] -> w541
              tunnel: [w556 w560] -> w540
              frame False {
                n222 = Unbundle By Name(w559) -> ("Axes Number"=w558:u8, "Axis 2: sp Position"=w557:dbl, "Axis 2: sp rot count"=w556:i32)
              }
              frame True {
                n223 = Unbundle By Name(w563) -> ("Axes Number"=w562:u8, "Axis 1: sp Position"=w561:dbl, "Axis 1: sp rot count"=w560:i32)
              }
            }
            n224 = Bundle By Name(cluster=w551, "SelfRef"=w548) -> (w552:T5)
            n225 = call "ANC350_MoveAbsolute.vi"("device handle"=w543, "axis no"=w542, "absoluteposition [µm/°/m°]"=w541, "rot count"=w540, "error in"=w539) -> ("error out"=w538:T9)  [unwired: 9 in, 1 out]
            n226 = call <vilib>:"Add State(s) to Queue__jki_lib_state_machine.vi"("State(s) in (\"\")"=w555) -> ("States Out"=w554:string)  [unwired: 14 in]
          }
          frame "Instrument: CapMeasure" {
            w575 = T8 {"Handle"=0, "Axes Number"=0, "Axis 1: sp Position"=0.0, "Axis 2: sp Position"=0.0, "Axis 1: sp rot count"=0, "Axis 2: sp rot count"=0, "Backward or Forward?"=FALSE, "Axis 1: Amplitude [V] "=0.0, "Axis 2: Amplitude [V] "=0.0, "Axis 1: DCLevel [V]"=0.0, "Axis 2: DCLevel [V]"=0.0, "Axis 1: Frequency [Hz]"=0, "Axis 2: Frequency [Hz]"=0, "Axis 1:\ncontrol mode"=enum."amplitude", "Axis 2:\ncontrol mode"=enum."amplitude", "axis 1:\nOutput"=FALSE, "axis 2:\nOutput 2"=FALSE, "axis 1:\nstop detection"=FALSE, "axis 2:\nstop detection"=FALSE, "axis 1:\nSingle Circle Mode"=FALSE, "axis 2:\nSingle Circle Mode"=FALSE, "axis 1: \nTarget GND"=FALSE, "axis 2: \nTarget GND"=FALSE}  # Inputs
            n227 = Unbundle By Name(w577) -> ("SelfRef"=w565:refnum<class "Inst.Attocube-3DR.lvclass">, "MessageToProcess.Message.Data"=w576:variant)
            n228 = call "Variant to LV Data.vim"("type"=w575, "JSON Data in"=w576) -> ("Data out"=w572:T8)  [unwired: 6 in, 3 out]
            n229 = Unbundle By Name(w572) -> ("Axes Number"=w573:u8)
            n230 = Equal?(x=w573, y=u8 1) -> (x = y?=w564:bool)
            n231 = Unbundle By Name(w565) -> ("handle"=w569:i32)
            n232 = case shown="False" w564 {
              tunnel: w572 -> [w589 w591]
              tunnel: [w588 w590] -> w568
              frame False {
                n233 = Unbundle By Name(w589) -> ("Axes Number"=w588:u8)
              }
              frame True {
                n234 = Unbundle By Name(w591) -> ("Axes Number"=w590:u8)
              }
            }
            n235 = call "ANC350_CapMeasure.vi"("error in"=w567, "axis no"=w568, "device handle"=w569) -> ("error out"=w566:T9, "Capacitance"=w571:i32)  [unwired: 2 in, 1 out]
            n236 = case shown="True" w564 {
              tunnel: w571 -> [w582 w585]
              tunnel: [w583 w587] -> w570
              tunnel: w565 -> [w584 w586]
              frame False {
                n237 = Bundle By Name(cluster=w584, "Axis 2: Capacitance"=w582) -> (w583:refnum<class "Inst.Attocube-3DR.lvclass">)
              }
              frame True {
                n238 = Bundle By Name(cluster=w586, "Axis 1: Capacitance"=w585) -> (w587:refnum<class "Inst.Attocube-3DR.lvclass">)
              }
            }
            n239 = Bundle By Name(cluster=w577, "SelfRef"=w570) -> (w578:T5)
            n240 = call <vilib>:"Add State(s) to Queue__jki_lib_state_machine.vi"("State(s) in (\"\")"=w581) -> ("States Out"=w580:string)  [unwired: 14 in]
          }
          frame "Instrument: StopDetection" {
            w602 = T8 {"Handle"=0, "Axes Number"=0, "Axis 1: sp Position"=0.0, "Axis 2: sp Position"=0.0, "Axis 1: sp rot count"=0, "Axis 2: sp rot count"=0, "Backward or Forward?"=FALSE, "Axis 1: Amplitude [V] "=0.0, "Axis 2: Amplitude [V] "=0.0, "Axis 1: DCLevel [V]"=0.0, "Axis 2: DCLevel [V]"=0.0, "Axis 1: Frequency [Hz]"=0, "Axis 2: Frequency [Hz]"=0, "Axis 1:\ncontrol mode"=enum."amplitude", "Axis 2:\ncontrol mode"=enum."amplitude", "axis 1:\nOutput"=FALSE, "axis 2:\nOutput 2"=FALSE, "axis 1:\nstop detection"=FALSE, "axis 2:\nstop detection"=FALSE, "axis 1:\nSingle Circle Mode"=FALSE, "axis 2:\nSingle Circle Mode"=FALSE, "axis 1: \nTarget GND"=FALSE, "axis 2: \nTarget GND"=FALSE}  # Inputs
            n241 = Unbundle By Name(w604) -> ("SelfRef"=w601:refnum<class "Inst.Attocube-3DR.lvclass">, "MessageToProcess.Message.Data"=w603:variant)
            n242 = call "Variant to LV Data.vim"("type"=w602, "JSON Data in"=w603) -> ("Data out"=w599:T8)  [unwired: 6 in, 3 out]
            n243 = Unbundle By Name(w599) -> ("Axes Number"=w598:u8)
            n244 = Equal?(x=w598, y=u8 1) -> (x = y?=w597:bool)
            n245 = Unbundle By Name(w601) -> ("handle"=w596:i32)
            n246 = case shown="True" w597 {
              tunnel: w599 -> [w611 w614]
              tunnel: [w610 w613] -> w595
              tunnel: [w609 w612] -> w592
              frame False {
                n247 = Unbundle By Name(w611) -> ("Axes Number"=w610:u8, "axis 2:\nstop detection"=w609:bool)
              }
              frame True {
                n248 = Unbundle By Name(w614) -> ("Axes Number"=w613:u8, "axis 1:\nstop detection"=w612:bool)
              }
            }
            n249 = Bundle By Name(cluster=w604, "SelfRef"=w601) -> (w605:T5)
            n250 = call "ANC350_StopDetection.vi"("error in"=w594, "enable"=w592, "axis no"=w595, "device handle"=w596) -> ("error out"=w593:T9)  [unwired: 2 in, 1 out]
            n251 = call <vilib>:"Add State(s) to Queue__jki_lib_state_machine.vi"("State(s) in (\"\")"=w608) -> ("States Out"=w607:string)  [unwired: 14 in]
          }
          frame "Instrument: SingleCircleMode" {
            w625 = T8 {"Handle"=0, "Axes Number"=0, "Axis 1: sp Position"=0.0, "Axis 2: sp Position"=0.0, "Axis 1: sp rot count"=0, "Axis 2: sp rot count"=0, "Backward or Forward?"=FALSE, "Axis 1: Amplitude [V] "=0.0, "Axis 2: Amplitude [V] "=0.0, "Axis 1: DCLevel [V]"=0.0, "Axis 2: DCLevel [V]"=0.0, "Axis 1: Frequency [Hz]"=0, "Axis 2: Frequency [Hz]"=0, "Axis 1:\ncontrol mode"=enum."amplitude", "Axis 2:\ncontrol mode"=enum."amplitude", "axis 1:\nOutput"=FALSE, "axis 2:\nOutput 2"=FALSE, "axis 1:\nstop detection"=FALSE, "axis 2:\nstop detection"=FALSE, "axis 1:\nSingle Circle Mode"=FALSE, "axis 2:\nSingle Circle Mode"=FALSE, "axis 1: \nTarget GND"=FALSE, "axis 2: \nTarget GND"=FALSE}  # Inputs
            n252 = Unbundle By Name(w627) -> ("SelfRef"=w624:refnum<class "Inst.Attocube-3DR.lvclass">, "MessageToProcess.Message.Data"=w626:variant)
            n253 = call "Variant to LV Data.vim"("type"=w625, "JSON Data in"=w626) -> ("Data out"=w622:T8)  [unwired: 6 in, 3 out]
            n254 = Unbundle By Name(w622) -> ("Axes Number"=w621:u8)
            n255 = Equal?(x=w621, y=u8 1) -> (x = y?=w620:bool)
            n256 = Unbundle By Name(w624) -> ("handle"=w619:i32)
            n257 = case shown="False" w620 {
              tunnel: w622 -> [w634 w637]
              tunnel: [w633 w636] -> w618
              tunnel: [w632 w635] -> w617
              frame False {
                n258 = Unbundle By Name(w634) -> ("Axes Number"=w633:u8, "axis 2:\nSingle Circle Mode"=w632:bool)
              }
              frame True {
                n259 = Unbundle By Name(w637) -> ("Axes Number"=w636:u8, "axis 1:\nSingle Circle Mode"=w635:bool)
              }
            }
            n260 = Bundle By Name(cluster=w627, "SelfRef"=w624) -> (w628:T5)
            n261 = call "ANC350_SingleCircleMode.vi"("error in"=w616, "enable"=w617, "axis no"=w618, "device handle"=w619) -> ("error out"=w615:T9)  [unwired: 2 in, 1 out]
            n262 = call <vilib>:"Add State(s) to Queue__jki_lib_state_machine.vi"("State(s) in (\"\")"=w631) -> ("States Out"=w630:string)  [unwired: 14 in]
          }
          frame "Instrument: SetTargetGround" {
            w648 = T8 {"Handle"=0, "Axes Number"=0, "Axis 1: sp Position"=0.0, "Axis 2: sp Position"=0.0, "Axis 1: sp rot count"=0, "Axis 2: sp rot count"=0, "Backward or Forward?"=FALSE, "Axis 1: Amplitude [V] "=0.0, "Axis 2: Amplitude [V] "=0.0, "Axis 1: DCLevel [V]"=0.0, "Axis 2: DCLevel [V]"=0.0, "Axis 1: Frequency [Hz]"=0, "Axis 2: Frequency [Hz]"=0, "Axis 1:\ncontrol mode"=enum."amplitude", "Axis 2:\ncontrol mode"=enum."amplitude", "axis 1:\nOutput"=FALSE, "axis 2:\nOutput 2"=FALSE, "axis 1:\nstop detection"=FALSE, "axis 2:\nstop detection"=FALSE, "axis 1:\nSingle Circle Mode"=FALSE, "axis 2:\nSingle Circle Mode"=FALSE, "axis 1: \nTarget GND"=FALSE, "axis 2: \nTarget GND"=FALSE}  # Inputs
            n263 = Unbundle By Name(w650) -> ("SelfRef"=w647:refnum<class "Inst.Attocube-3DR.lvclass">, "MessageToProcess.Message.Data"=w649:variant)
            n264 = call "Variant to LV Data.vim"("type"=w648, "JSON Data in"=w649) -> ("Data out"=w645:T8)  [unwired: 6 in, 3 out]
            n265 = Unbundle By Name(w645) -> ("Axes Number"=w644:u8)
            n266 = Equal?(x=w644, y=u8 1) -> (x = y?=w643:bool)
            n267 = Unbundle By Name(w647) -> ("handle"=w640:i32)
            n268 = case shown="True" w643 {
              tunnel: w645 -> [w657 w660]
              tunnel: [w656 w659] -> w639
              tunnel: [w655 w658] -> w638
              frame False {
                n269 = Unbundle By Name(w657) -> ("Axes Number"=w656:u8, "axis 2: \nTarget GND"=w655:bool)
              }
              frame True {
                n270 = Unbundle By Name(w660) -> ("Axes Number"=w659:u8, "axis 1: \nTarget GND"=w658:bool)
              }
            }
            n271 = Bundle By Name(cluster=w650, "SelfRef"=w647) -> (w651:T5)
            n272 = call "ANC350_SetTargetGround.vi"("error in"=w642, "PositionerAcIn"=w638, "axis no"=w639, "device handle"=w640) -> ("error out"=w641:T9)  [unwired: 2 in, 1 out]
            n273 = call <vilib>:"Add State(s) to Queue__jki_lib_state_machine.vi"("State(s) in (\"\")"=w654) -> ("States Out"=w653:string)  [unwired: 14 in]
          }
          frame "Instrument: Open Hardware" {
            n274 = Unbundle By Name(w665) -> ("SelfRef"=w664:refnum<class "Inst.Attocube-3DR.lvclass">)
            n275 = call-dynamic "Open Hardware.vi"("error in (no error)"=w661, "Inst.Attocube-3DR in"=w664) -> ("error out"=w662:errorcluster, "Inst.Attocube-3DR out"=w663:refnum<class "Inst.Attocube-3DR.lvclass">)  [unwired: 8 in]
            n276 = Bundle By Name(cluster=w665, "SelfRef"=w663) -> (w666:T5)
            n277 = call <vilib>:"Add State(s) to Queue__jki_lib_state_machine.vi"("State(s) in (\"\")"=w669) -> ("States Out"=w668:string)  [unwired: 14 in]
          }
          frame "Instrument: Close Hardware" {
            n278 = Unbundle By Name(w674) -> ("SelfRef"=w673:refnum<class "Inst.Attocube-3DR.lvclass">)
            n279 = call-dynamic "Close Hardware.vi"("error in (no error)"=w670, "Inst.Attocube-3DR in"=w673) -> ("error out"=w671:errorcluster, "Inst.Attocube-3DR out"=w672:refnum<class "Inst.Attocube-3DR.lvclass">)  [unwired: 8 in]
            n280 = Bundle By Name(cluster=w674, "SelfRef"=w672) -> (w675:T5)
            n281 = call <vilib>:"Add State(s) to Queue__jki_lib_state_machine.vi"("State(s) in (\"\")"=w678) -> ("States Out"=w677:string)  [unwired: 14 in]
          }
          frame "Instrument: GetAll" {
            # "communicate with\nhardware"
            n282 = Unbundle By Name(w680) -> ("SelfRef"=w679:refnum<class "Inst.Attocube-3DR.lvclass">, "MessageToProcess.Message.ID"=w681:string)
            n283 = call "Inst.Attocube-3DR.GetAllData.vi"("error in (no error)"=w688, "Inst.Attocube-3DR in"=w679) -> ("error out"=w684:errorcluster, "Data out"=w683:variant, "Inst.Attocube-3DR out"=w687:refnum<class "Inst.Attocube-3DR.lvclass">)  [unwired: 7 in]
            n284 = Empty String/Path?(string/path=w683) -> (empty?=w682:bool)
            n285 = case shown="False" w682 {
              tunnel: w687 -> [w699 w701]
              tunnel: [w698 w701] -> w686
              tunnel: [w697 w700] -> w685
              tunnel: w683 -> [w694 _]
              tunnel: w684 -> [w693 w700]
              tunnel: w681 -> [w695 _]
              frame False {
                # "send data to\ninstrument:process.vi"
                n286 = call <userlib>:"Instrument.MessageToProcess.vi"("ID"=w695, "error in (no error)"=w693, "Data"=w694, "Command"="Set GetAll", "Instrument"=w699) -> ("error out"=w697:errorcluster, "Instrument out"=w698:refnum<class "Inst.Attocube-3DR.lvclass">)  [unwired: 5 in]
              }
              frame True {
              }
            }
            n287 = Bundle By Name(cluster=w680, "SelfRef"=w686) -> (w689:T5)
            n288 = call <vilib>:"Add State(s) to Queue__jki_lib_state_machine.vi"("State(s) in (\"\")"=w692) -> ("States Out"=w691:string)  [unwired: 14 in]
          }
          frame "---------- Sequence ----------" {
            n289 = call <vilib>:"Add State(s) to Queue__jki_lib_state_machine.vi"("State(s) in (\"\")"=w706) -> ("States Out"=w705:string)  [unwired: 14 in]
          }
          frame "Sequence: Status" {
            # "Sequence: Status\n(Use this frame to pass the status to the UI, this VI's UI, etc)"
            n290 = call <vilib>:"Add State(s) to Queue__jki_lib_state_machine.vi"("State(s) in (\"\")"=w712) -> ("States Out"=w711:string)  [unwired: 14 in]
            "Status" <- w707
          }
          frame "Sequence: Wait" {
            # "Sequence: Wait\n(Non-Blocking Wait)"
            # "F = repeat this state. wait\nT = go to next state. don't wait"
            n291 = Unbundle By Name(w721) -> ("Running Step"=w714:i32)
            n292 = call <userlib>:"Wait Logic.vi"("error in (no error)"=w717, "Time"=w715) -> ("error out"=w716:errorcluster, "Status String"=w713:string, "Trigger"=w718:bool)  [unwired: 6 in, 1 out]
            n293 = Increment(x=w714) -> (x+1=w728:i32)
            n294 = Select(t=w728, s=w718, f=w714) -> (s? t:f=w719:i32)
            n295 = Select(t=u32 0, s=w718, f=u32 100 ("milliseconds to wait")) -> (s? t:f=w725:u32)
            n296 = call <userlib>:"Wait (ms)__ogtk.vi"("error in (no error)"=w716, "milliseconds to wait"=w725) -> ("error out"=w723:errorcluster)  [unwired: 8 in, 1 out]
            n297 = Bundle By Name(cluster=w721, "Running Step"=w719) -> (w720:T5)
            n298 = call <vilib>:"Build State String with Arguments__JKI_lib_State_Machine.vi"("Arguments (\"\")"=w713, "State"="Sequence: Status") -> ("State with Arguments"=w722:string)  [unwired: 4 in]
            n299 = call <vilib>:"Add State(s) to Queue__jki_lib_state_machine.vi"("State(s) in Front (\"\")"=w722, "State(s) in (\"\")"=w731) -> ("States Out"=w730:string)  [unwired: 13 in]
          }
        }
      }
    }
    frame Error {
    }
  }
  n300 = call-parent "Process.vi"("error in"=w5, "Instrument"=w4) -> ("error out"=w2:errorcluster, "Instrument out"=→"Inst.Attocube-3DR out":refnum<class "Inst.Attocube-3DR.lvclass">)  [unwired: 8 in]
  n301 = Merge Errors(w2, w1) -> (→"error out":errorcluster)
  n302 = call "ANC350_StaticAmplitude.vi"() -> ()  [unwired: 6 in, 2 out]
